vi "OTECCM-SECCM-Master-Program.vi"() -> ()   [LabVIEW 2016]
uses:
  SpectroElectroChem_1Electrode_caseEnum.ctl
  <vilib>/Utility/error.llb/DialogType.ctl
  <vilib>/DAQmx/write.llb/DAQmx Write (Analog 1D DBL 1Chan NSamp).vi
  <vilib>/DAQmx/write.llb/DAQmx Write (Analog DBL 1Chan 1Samp).vi
  <vilib>/DAQmx/read.llb/DAQmx Read (Analog 2D DBL NChan NSamp).vi
  <vilib>/Analysis/baseanly.llb/Mean (DBL).vi
  <vilib>/DAQmx/create/channels.llb/DAQmx Create Channel (AI-Voltage-Basic).vi
  <vilib>/DAQmx/configure/timing.llb/DAQmx Timing (Sample Clock).vi
  <vilib>/DAQmx/create/channels.llb/DAQmx Create Channel (AO-Voltage-Basic).vi
  <vilib>/DAQmx/miscellaneous.llb/DAQmx Fill In Error Info.vi
  <vilib>/Utility/file.llb/Write Delimited Spreadsheet (DBL).vi
  <vilib>/DAQmx/configure/trigger.llb/DAQmx Start Trigger (Digital Edge).vi
  <vilib>/Utility/file.llb/Write Delimited Spreadsheet (I64).vi
  <vilib>/DAQmx/configure/trigger.llb/DAQmx Start Trigger (None).vi
  <vilib>/measure/NI_MABase.lvlib
  <vilib>/Analysis/NI_AALBase.lvlib
  <resource>/objmgr/daqmx.rc
panel:
  out "dy":dbl
  out "ny":dbl
  out "dx":dbl
  out "nx":dbl
  in  "Clear POI":bool
  out "Points of Interest":dbl[][](array[numeric])
  out "Piezo Velocity / um/s":dbl[](array[numeric]) format="%.6f"
  out "Stopped":bool
  out "Piezo z":dbl
  out "Piezo y":dbl
  out "Piezo x":dbl
  out "Econtrol":refnum<k21>
  out "i tip":dbl(graph)
  out "E-Chem Data Point":i32
  in  "Stop Action":bool
  out "Acquisition Progress":u8(slide) scale=0.0..100.0
  out "Stage Task":refnum<k21>
  out "CCD Image":i32[][](graph)
  out "Background":i32[][](array[numeric])
  in  "Tab Control":T1(tab)
  in  "Tip Filter (Hz)":u16(ring) items=["100", "300", "1K", "3K", "10K"]
  in  "Tip Gain (mV/pA)":dbl(ring)=1.0 items=["0.1"=0.1, "0.2"=0.2, "0.5"=0.5, "1"=1.0, "2"=2.0, "5"=5.0, "10"=10.0, "20"=20.0]
  in  "Cycles":dbl
  in  "Start CV":bool
  in  "Initial E / V":dbl
  in  "Final E / V":dbl
  in  "v / mV/s":dbl
  out "Tip Voltammogram":cluster{dbl[], dbl[]}(graph)
  in  "Setpoint Direction":u16(ring) items=["Positive", "Negative"]
  in  "Setpoint / A":dbl
  out "Tip Approach Curve":cluster{dbl[], dbl[]}(graph)
  in  "Initial z":dbl
  in  "Final z":dbl
  in  "z Res.":dbl
  in  "t / pt / s":dbl
  in  "Start Approach Curve":bool
  in  "Stop Approach \nCurve":bool
  in  "Stop TarSECCM":bool
  in  "Targeted SECCM":bool
  in  "Retraction / um":dbl=3.0
  in  "Approach Set / A":dbl=3e-12
  in  "E Approach / V":dbl=-0.75
  in  "t / s/pt":dbl=0.002
  in  "z Res. / um":dbl=0.004
  out "Height Image":dbl[][](graph)
  out "SECM Image":dbl[][](graph)
  in  "xi / um":dbl
  in  "xf / um":dbl=20.0
  in  "xy Res. / um":dbl=0.5
  in  "yi / um":dbl
  in  "yf / um":dbl=20.0
  in  "Start SECM Image":bool
  in  "Stop SECM Image":bool
  out "Tip Voltammogram 2":cluster{dbl[], dbl[]}(graph)
  out "Tip Approach Curve 2":cluster{dbl[], dbl[]}(graph)
  in  "SECCM SP Dir":u16(ring)=1 items=["Positive", "Negative"]
  in  "CV v / mV/s":dbl=2000.0
  in  "CV Ef / V":dbl=0.5
  in  "CV Ei / V":dbl=-0.75
  in  "CV Cycles":dbl=0.5
  in  "Clear Background":bool
  in  "Aquire Background":bool
  out "xpixels":i32
  out "ypixels":i32
  in  "HSS (MHz)":i32(ring) items=["3.000000", "1.000000", "0.050000"]
  in  "VSS (us)":i32(ring) items=["4.880000", "9.680000", "19.280001", "38.470001", "57.680000"]
  in  "Exp. Time":sgl=0.1 format="%.2f"
  in  "# of Acc.":i32=1
  in  "EM Gain":i32=1
  in  "Binning":i32=1
  out "Cycle Time":sgl format="%.2f"
  out "Actual Temp.":i32
  in  "Background \nFrames":i32=10
  in  "Slit Width (um)":dbl=50.0
  in  "Center Wavelength (nm)":dbl
  out "Left":dbl
  out "Center":dbl
  out "Right":dbl
  in  "Grating":u16(ring) items=["1", "2", "3"]
  out "Lines/mm":i32=300
  in  "x Step (um)":dbl=0.25
  in  "Final x (um)":dbl=20.0
  in  "Initial x (um)":dbl
  out "Total Intensity":i32[][](graph)
  in  "Rest x (um)":dbl
  in  "Get HSI":bool
  in  "Delta":dbl=0.9267
  in  "Gamma":dbl=-0.064
  in  "Beta":dbl=0.0061
  in  "Alpha":dbl=1.1435
  in  "y":dbl
  in  "y'":dbl
  in  "x'":dbl
  in  "x":dbl
  out "bx":dbl
  out "by":dbl
  in  "Sample z":dbl
  in  "Sample y":dbl
  in  "Sample x":dbl
  out "Piezo Axes":string[](array[string])
  out "Resting?":bool
  out "Monitor":refnum<k21>
  out "Etip":dbl(graph)
  in  "WE Rest E (V)":dbl=-0.75
  out "Cell On?":bool
  out "Connected?":bool
  in  "Shutdown":bool
  # "HSI"
  # "SECCM"
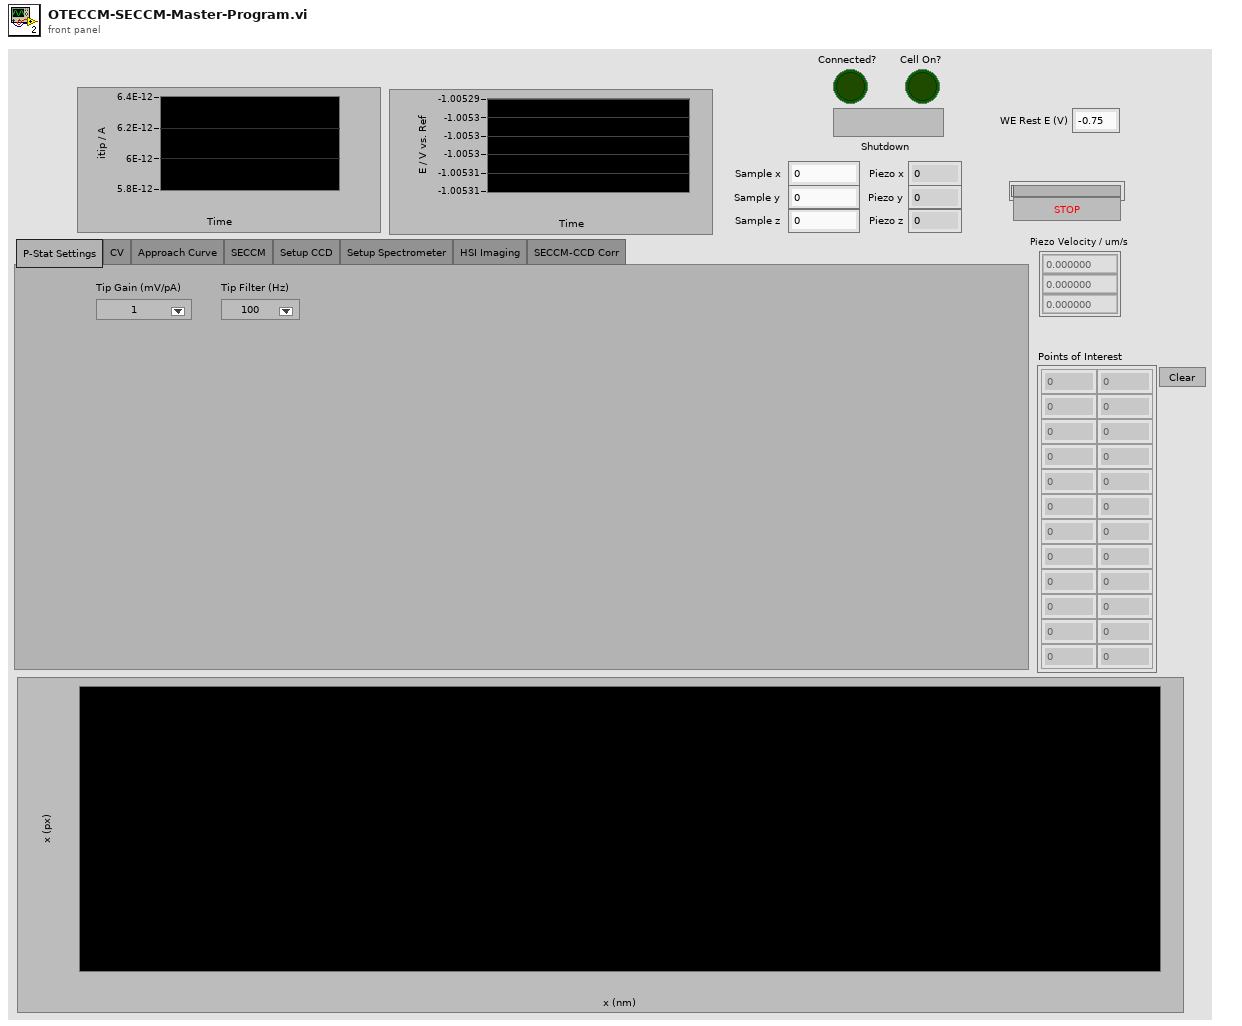
[diagram p1: front panel]
types:
  T1 = enum32{"P-Stat Settings", "CV", "Approach Curve", "SECCM", "Setup CCD", "Setup Spectrometer", "HSI Imaging", "SECCM-CCD Corr"}
  T2 = typedef "SpectroElectroChem_1Electrode_caseEnum.ctl" = enum16{"Initialize", "Rest", "Set Range", "Change Grating", "Move Grating", "Adjust Slit", "Setup CCD", "Acquire CCD BG", "Clear CCD BG", "Move Stage", "Cell On", "Cell Off", "Set E", "Move Piezo", "Acquire HSI", "Approach Curve", "Acquire SECCM Image", "Targeted SECCM", "Acquire CV", "Shutdown"}
  T3 = typedef "DialogType.ctl" = u16
  T4 = typedef "LVPoint32TypeDef.ctl" = cluster{"Horizontal":i32, "Vertical":i32}
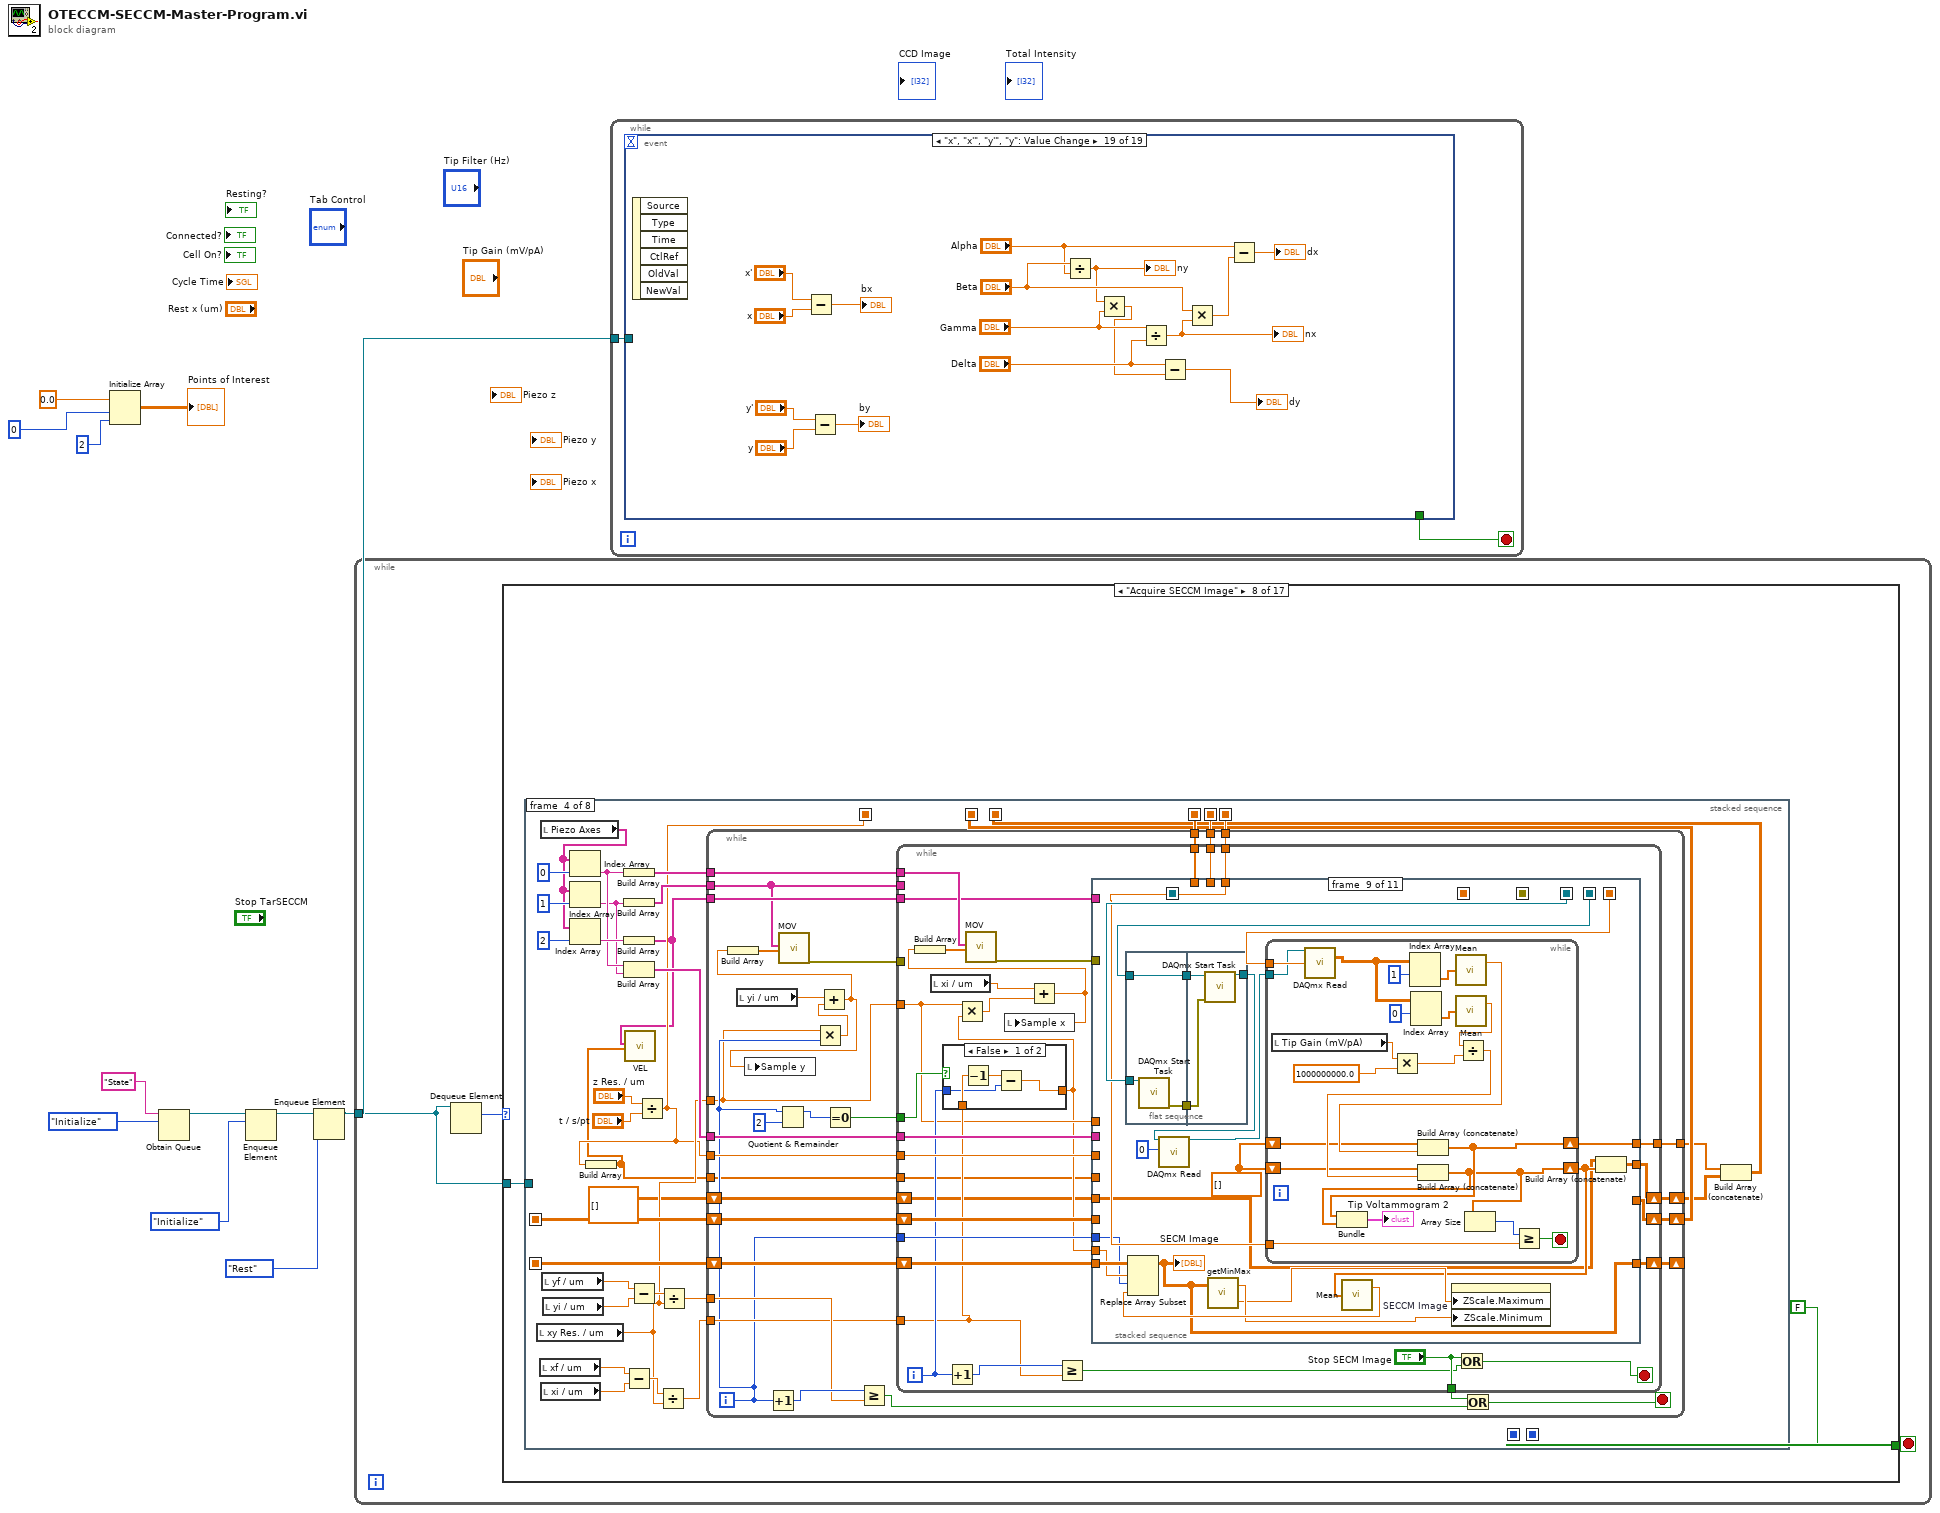
[diagram p0: block diagram]
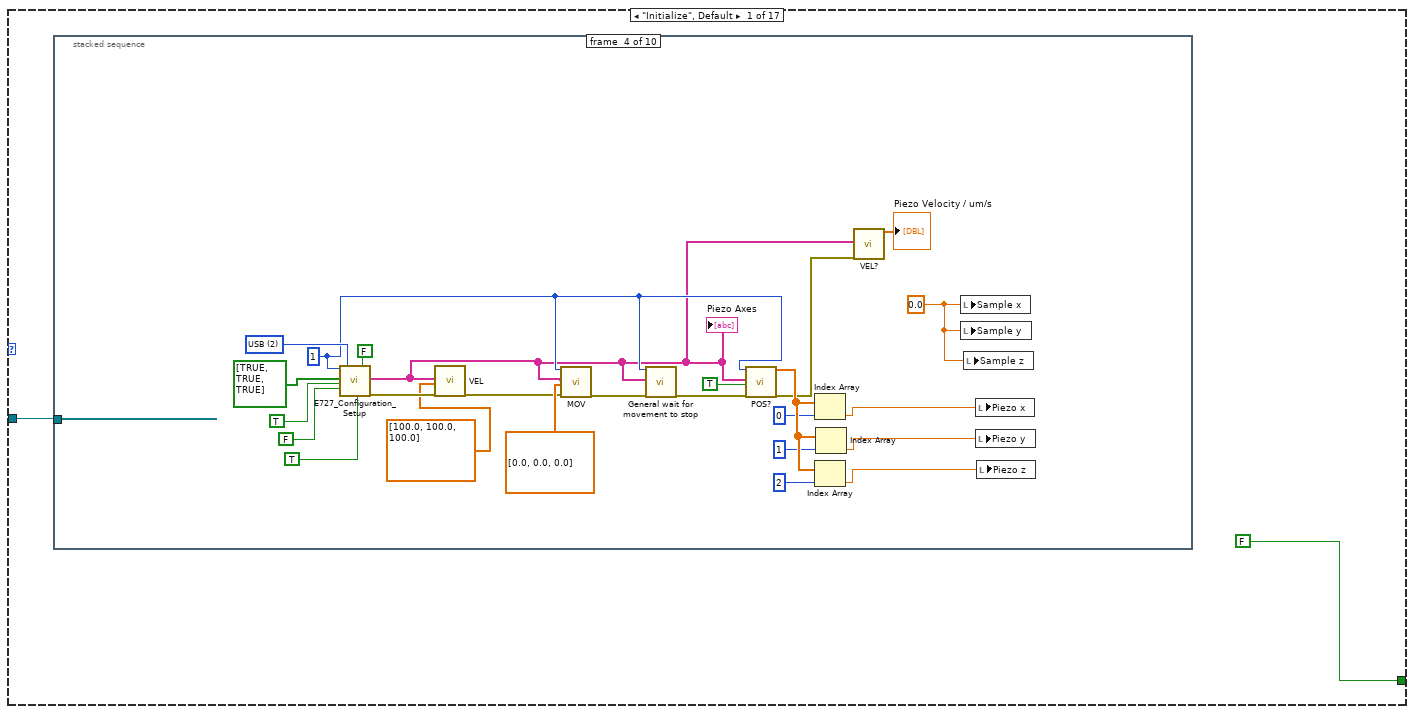
[diagram p2: hidden frame]
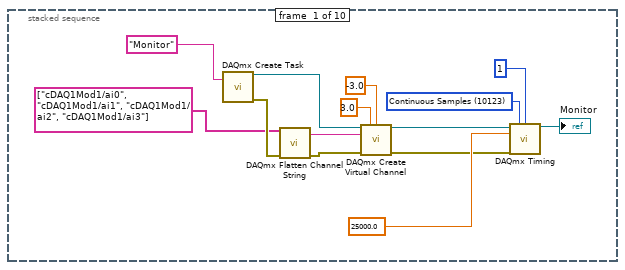
[diagram p3: hidden frame]
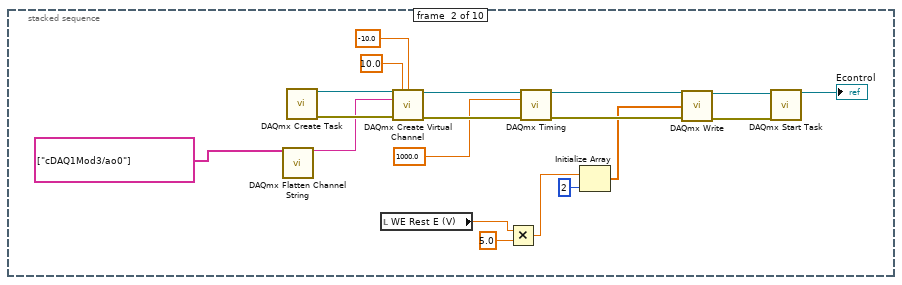
[diagram p4: hidden frame]
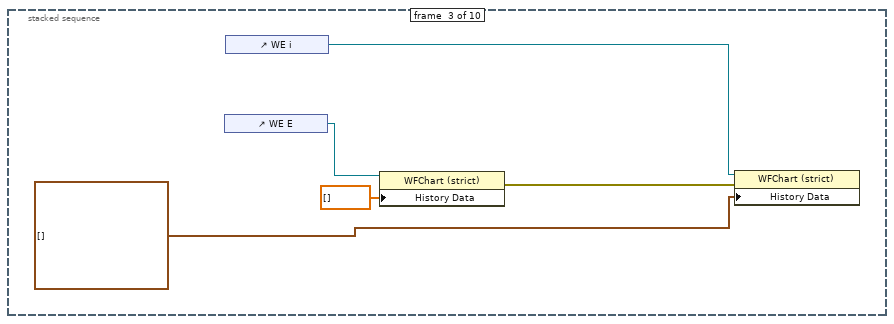
[diagram p5: hidden frame]
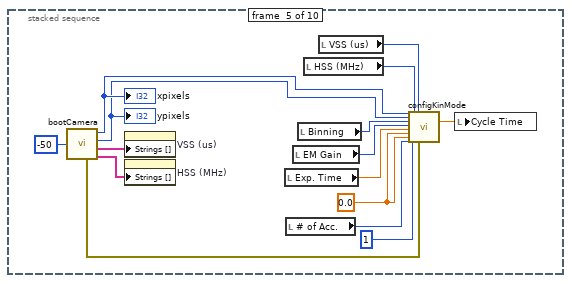
[diagram p6: hidden frame]
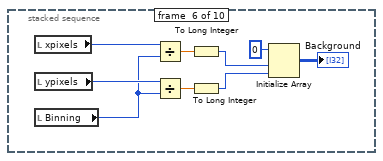
[diagram p7: hidden frame]
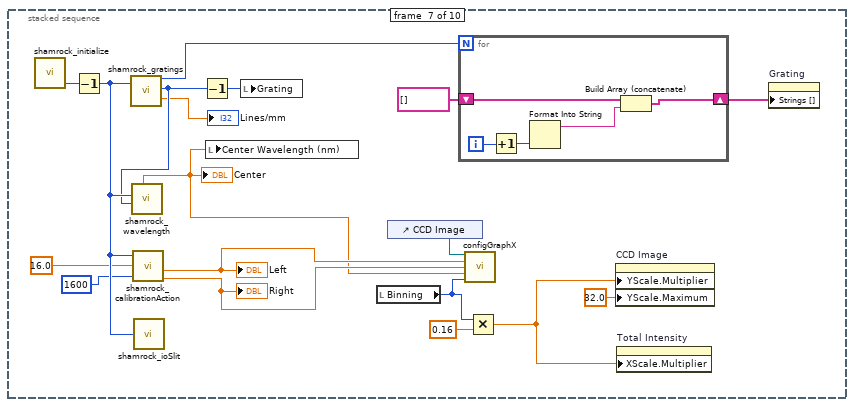
[diagram p8: hidden frame]
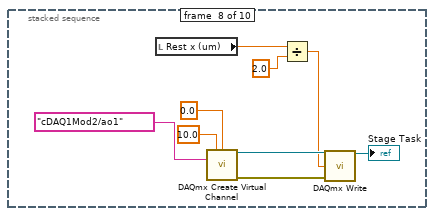
[diagram p9: hidden frame]
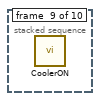
[diagram p10: hidden frame]
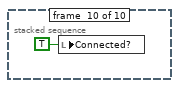
[diagram p11: hidden frame]
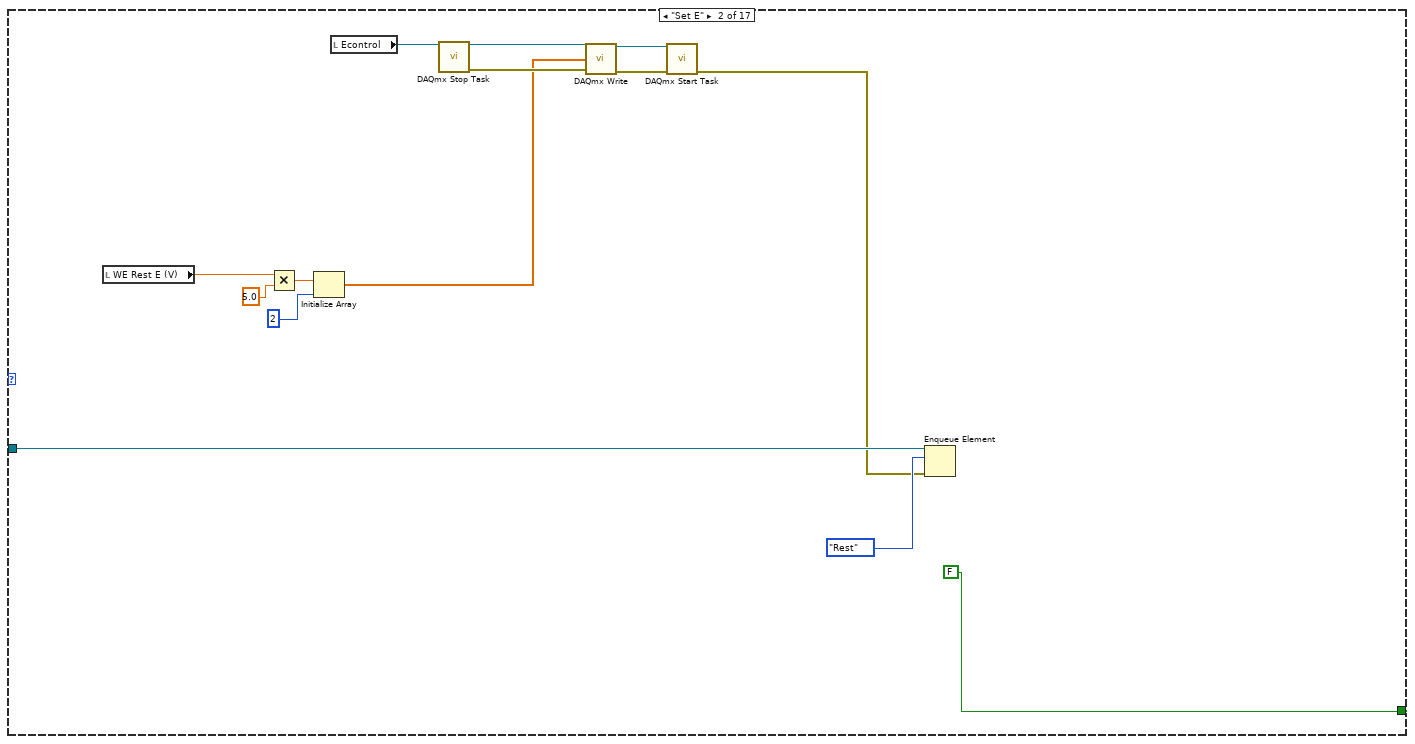
[diagram p12: hidden frame]
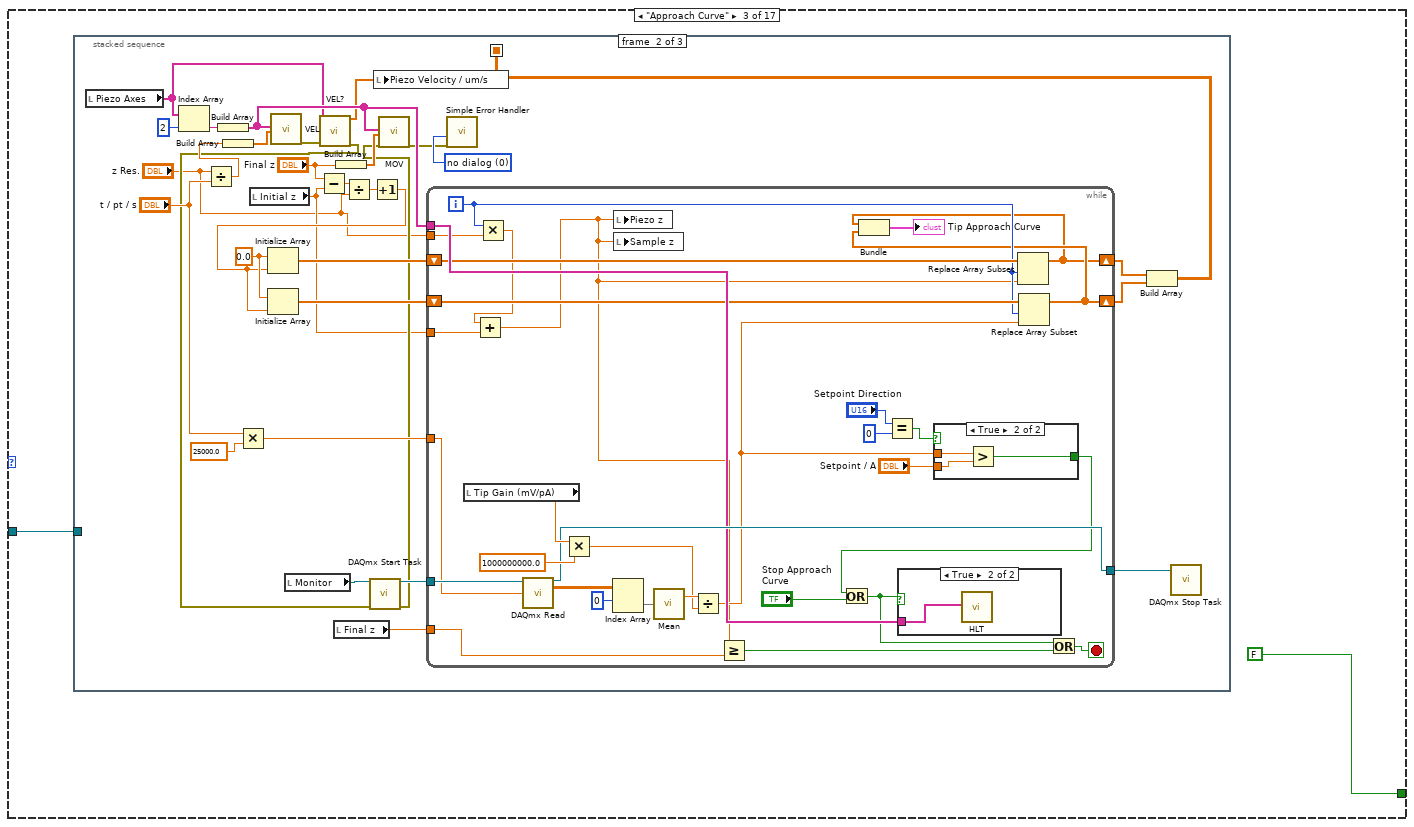
[diagram p13: hidden frame]
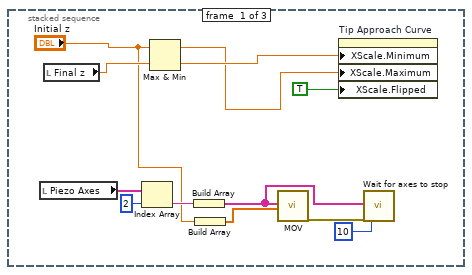
[diagram p14: hidden frame]
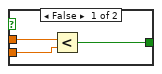
[diagram p15: hidden frame]
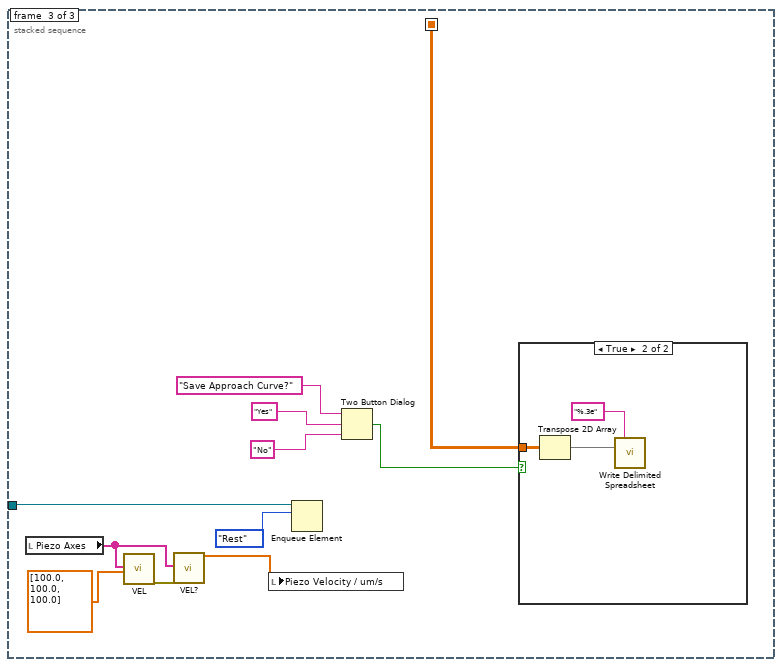
[diagram p17: hidden frame]
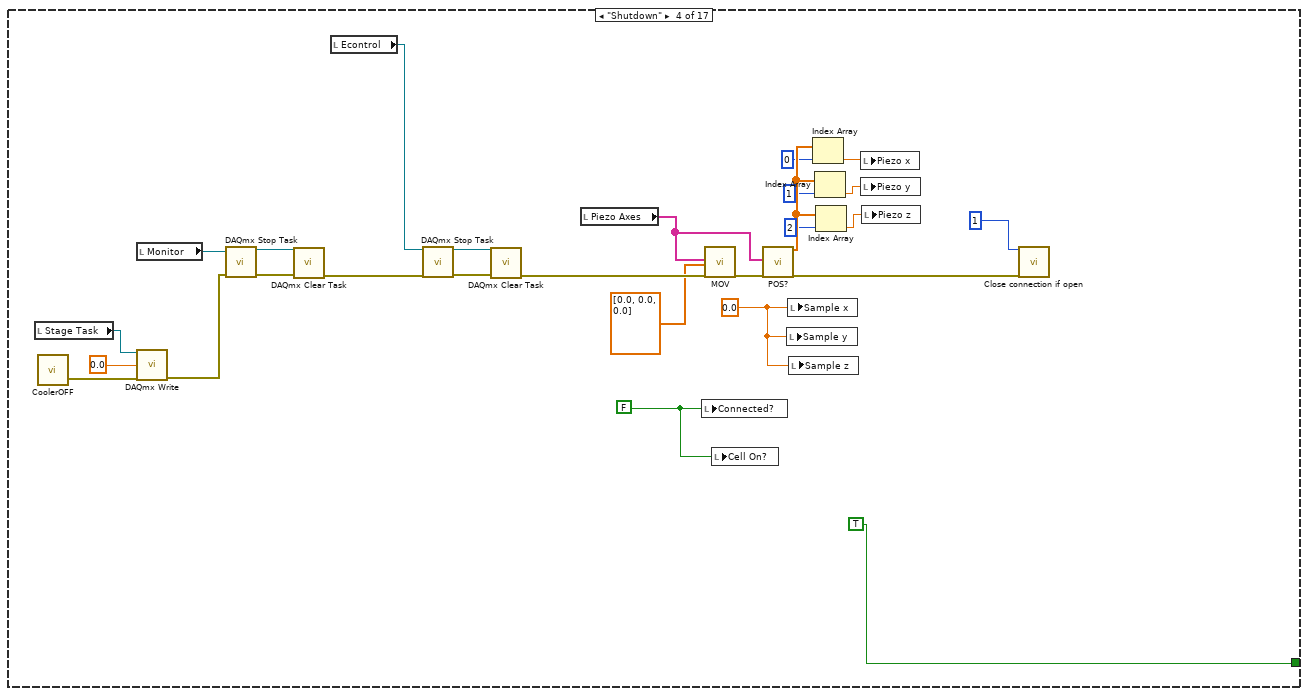
[diagram p19: hidden frame]
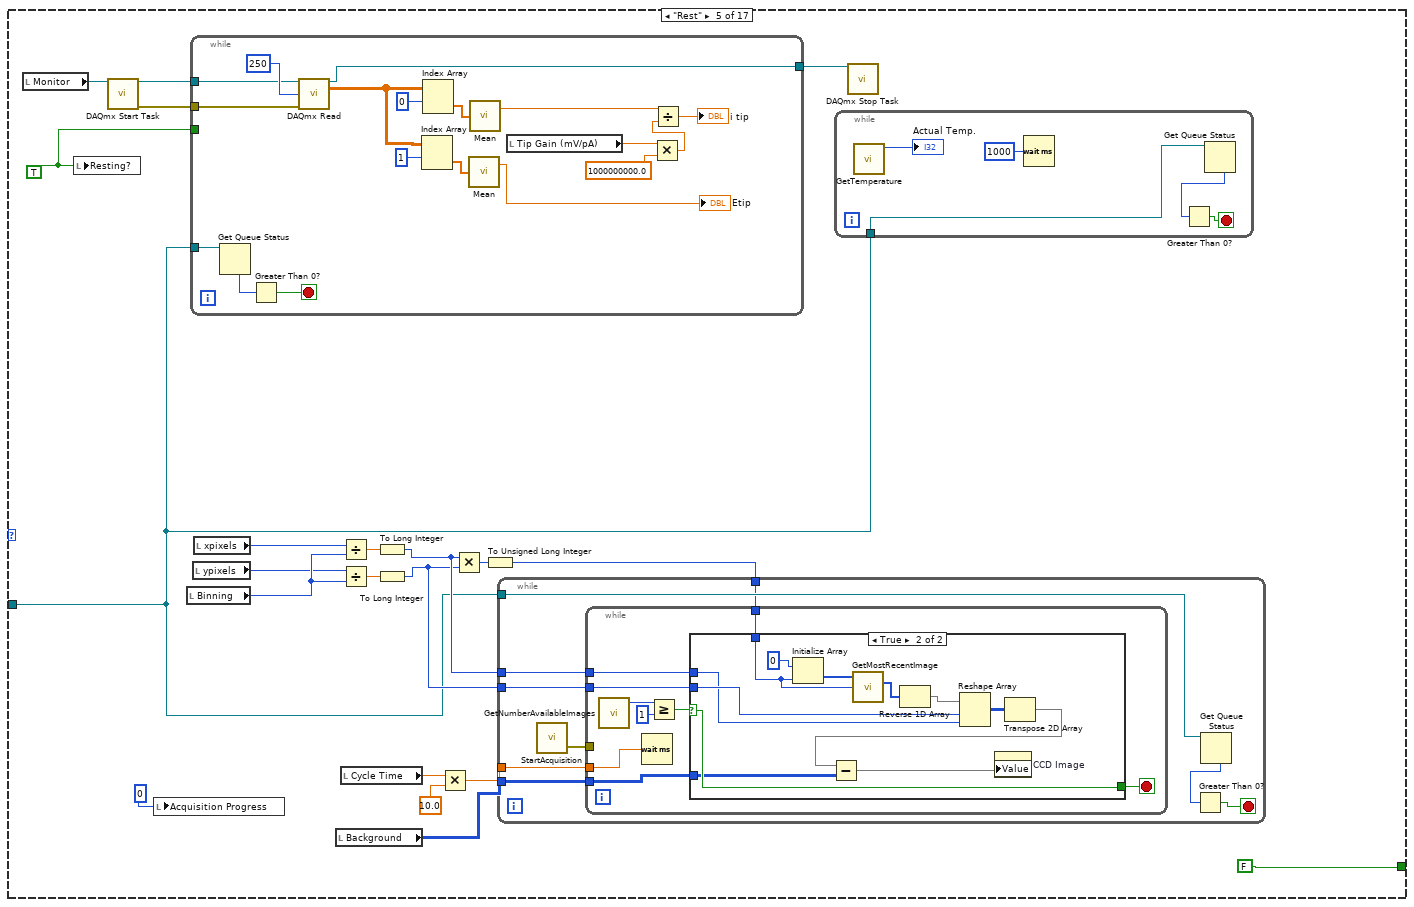
[diagram p20: hidden frame]
diagram:
  n1 = Initialize Array(0.0 ("element"), 0 ("dimension size"), 2 ("dimension size")) -> (→"Points of Interest":dbl[][])
  n2 = Obtain Queue(name (unnamed)="State", element data type=SpectroElectroChem_1Electrode_caseEnum."Initialize") -> (queue out=w10:refnum<queue>)  [unwired: 3 in, 2 out]
  n3 = Enqueue Element(queue=w10, element=SpectroElectroChem_1Electrode_caseEnum."Initialize") -> (queue out=w8:refnum<queue>)  [unwired: 2 in, 2 out]
  n4 = Enqueue Element(queue=w8, element=SpectroElectroChem_1Electrode_caseEnum."Rest") -> (queue out=w6:refnum<queue>)  [unwired: 2 in, 2 out]
  n5 = while {
    tunnel: w6 -> [w13]
    stop <- w14 stop-if-true
    n6 = Dequeue Element(queue=w13) -> (element=w12:T2)  [unwired: 2 in, 3 out]
    n7 = case shown="\"Acquire SECCM Image\"" w12 {
      tunnel: [FALSE FALSE FALSE TRUE FALSE FALSE FALSE FALSE FALSE FALSE FALSE FALSE FALSE FALSE FALSE FALSE FALSE] -> w14
      tunnel: w13 -> [w15 w143 w151 _ w279 w352 w381 w578 w1010 w1033 w1055 w1079 w1103 w1169 _ w1190 w1313]
      frame "Initialize", Default {
        n8 = stacked-sequence {
          tunnel: w15 -> [_ _ _ _ _ _ _ _ _ _]
          frame #0 {
            w21 = 10123 items=["Finite Samples"=10178, "Continuous Samples"=10123, "Hardware Timed Single Point"=12522] ("sample mode")
            n9 = call <vilib>:"DAQmx Create Task.vi"("new task name"="Monitor") -> ("task out"=w26:refnum<k21>, "error out"=w27:errorcluster)  [unwired: 13 in]
            n10 = call <vilib>:"DAQmx Flatten Channel String.vi"("names in"=tag[] ["cDAQ1Mod1/ai0", "cDAQ1Mod1/ai1", "cDAQ1Mod1/ai2", "cDAQ1Mod1/ai3"] ("physical channels"), "error in"=w27) -> ("names out"=w29:string, "error out"=w28:errorcluster)  [unwired: 12 in]
            n11 = call-poly <vilib>:"DAQmx Create Virtual Channel.vi"("task in"=w26, "maximum value"=3.0, "minimum value"=-3.0, "physical channels"=w29, "error in"=w28) -> ("task out"=w24:refnum<k21>, "error out"=w22:errorcluster)  [unwired: 9 in]
            n12 = call-poly <vilib>:"DAQmx Timing.vi"("task/channels in"=w24, "sample mode"=w21, "samples per channel"=1, "rate"=25000.0, "error in"=w22) -> ("task out"=→"Monitor":refnum<k21>)  [unwired: 9 in, 1 out]
          }
          frame #1 {
            n13 = call <vilib>:"DAQmx Flatten Channel String.vi"("names in"=tag[] ["cDAQ1Mod3/ao0"] ("physical channels")) -> ("names out"=w33:string)  [unwired: 13 in, 1 out]
            n14 = call <vilib>:"DAQmx Create Task.vi"() -> ("task out"=w49:refnum<k21>, "error out"=w43:errorcluster)  [unwired: 14 in]
            n15 = local read "WE Rest E (V)"() -> (w32:dbl)
            n16 = call-poly <vilib>:"DAQmx Create Virtual Channel.vi"("task in"=w49, "maximum value"=10.0, "minimum value"=-10.0, "physical channels"=w33, "error in"=w43) -> ("task out"=w48:refnum<k21>, "error out"=w42:errorcluster)  [unwired: 9 in]
            n17 = Multiply(x=w32, y=5.0) -> (x*y=w35:dbl)
            n18 = call-poly <vilib>:"DAQmx Timing.vi"("task/channels in"=w48, "rate"=1000.0, "error in"=w42) -> ("task out"=w47:refnum<k21>, "error out"=w41:errorcluster)  [unwired: 11 in]
            n19 = Initialize Array(w35, 2 ("dimension size")) -> (w31:dbl[])
            n20 = call-poly <vilib>:"DAQmx Write.vi"("task/channels in"=w47, "data"=w31, "error in"=w41) -> ("task out"=w46:refnum<k21>, "error out"=w40:errorcluster)  [unwired: 10 in, 1 out]
            n21 = call <vilib>:"DAQmx Start Task.vi"("task/channels in"=w46, "error in"=w40) -> ("task out"=→"Econtrol":refnum<k21>)  [unwired: 12 in, 1 out]
          }
          frame #2 {
            n22 = control-ref of="WE E"() -> (w54:refnum<vi>)
            n23 = control-ref of="WE i"() -> (w52:refnum<vi>)
            n24 = property on="Property Node" class="WFChart (strict)"(reference=w54, "History Data"=dbl[] []) -> (error out=w51:errorcluster)  [unwired: 1 in, 1 out]
            n25 = property on="Property Node" class="WFChart (strict)"(reference=w52, error in=w51, "History Data"=waveform(dbl)[] []) -> ()  [unwired: 2 out]
          }
          frame #3 {
            w55 = 0.0 ("Sample x")
            w62 = 1 ("System no.")
            w79 = u16 2 items=["RS232", "TCP/IP", "USB"] ("Interface")
            n26 = call "E727_Configuration_Setup.vi"("System no."=w62, "Are stages connected?"=bool[] [TRUE, TRUE, TRUE], "Change servo status to ON?"=TRUE, "Perform autozero?"=FALSE, "Interface"=w79, "Stop wave generator\noutput (if any)"=TRUE ("Stop wave generator\noutput (if any)"), "Move to middle?"=FALSE) -> ("All conn. axes"=w58:string[], "error out"=w61:errorcluster)  [unwired: 8 in, 3 out]
            "Piezo Axes" <- w58
            n27 = call "VEL.vi"("Axes to set"=w58, "Velocity values"=dbl[] [100.0, 100.0, 100.0] ("Position values"), "error in"=w61) -> ("error out"=w60:errorcluster)  [unwired: 15 in, 1 out]
            n28 = call "MOV.vi"("System no."=w62, "Axes to move"=w58, "Position values"=dbl[] [0.0, 0.0, 0.0], "error in"=w60) -> ("error out"=w71:errorcluster)  [unwired: 15 in]
            n29 = call "General wait for movement to stop.vi"("System no."=w62, "Axes to wait for"=w58, "error in"=w71) -> ("error out"=w70:errorcluster)  [unwired: 15 in, 1 out]
            n30 = call "POS?.vi"("System no."=w62, "Axes to query"=w58, "All axes?"=TRUE, "error in"=w70) -> ("Position"=w69:dbl[], "error out"=w57:errorcluster)  [unwired: 14 in]
            n31 = Index Array(array=w69, index=0) -> (element=w65:dbl)
            n32 = Index Array(array=w69, index=2) -> (element=w63:dbl)
            n33 = Index Array(array=w69, index=1) -> (element=w64:dbl)
            n34 = call "VEL?.vi"("Axes to query"=w58, "error in"=w57) -> ("Velocity"=→"Piezo Velocity / um/s":dbl[])  [unwired: 16 in, 1 out]
            n35 = local write "Sample x"(w55) -> ()
            n36 = local write "Sample y"(w55) -> ()
            n37 = local write "Sample z"(w55) -> ()
            n38 = local write "Piezo x"(w65) -> ()
            n39 = local write "Piezo y"(w64) -> ()
            n40 = local write "Piezo z"(w63) -> ()
          }
          frame #4 {
            w86 = sgl 0.0 ("Acc. Cycle Time")
            n41 = call "bootCamera.vi"("Target Temp"=-50) -> ("xpixels"=w81:i32, "ypixels"=w80:i32, "error out"=w83:errorcluster, "VSS"=w93:string[], "HSS"=w92:string[])  [unwired: 5 in]
            "xpixels" <- w81
            "ypixels" <- w80
            n42 = property on="VSS (us)" class="Ring (strict)"("Strings []"=w93) -> ()  [unwired: 2 in, 2 out]
            n43 = property on="HSS (MHz)" class="Ring (strict)"("Strings []"=w92) -> ()  [unwired: 2 in, 2 out]
            n44 = local read "Exp. Time"() -> (w87:sgl)
            n45 = local read "# of Acc."() -> (w85:i32)
            n46 = local read "EM Gain"() -> (w88:i32)
            n47 = local read "Binning"() -> (w89:i32)
            n48 = local read "HSS (MHz)"() -> (w90:i32)
            n49 = local read "VSS (us)"() -> (w91:i32)
            n50 = call "configKinMode.vi"("X Pixels"=w81, "Y Pixels"=w80, "Binning"=w89, "EM Gain"=w88, "Exp. Time"=w87, "Acc. Cycle Time"=w86, "Kin. Cycle Time"=w86, "# of Acc."=w85, "HSS"=w90, "# of Scans"=1, "VSS"=w91, "error in (no error)"=w83) -> ("Actual Kin. Cycle Time"=w82:sgl)  [unwired: 12 in, 3 out]
            n51 = local write "Cycle Time"(w82) -> ()
          }
          frame #5 {
            n52 = local read "xpixels"() -> (w97:i32)
            n53 = local read "ypixels"() -> (w96:i32)
            n54 = local read "Binning"() -> (w95:i32)
            n55 = Divide(x=w97, y=w95) -> (x/y=w103:dbl)
            n56 = Divide(x=w96, y=w95) -> (x/y=w102:dbl)
            n57 = To Long Integer(number=w103) -> (32bit integer=w100:i32)
            n58 = To Long Integer(number=w102) -> (32bit integer=w99:i32)
            n59 = Initialize Array(0 ("element"), w100, w99) -> (→"Background":i32[][])
          }
          frame #6 {
            n60 = call "shamrock_initialize.vi"() -> ("No of devices"=w121:i32)  [unwired: 1 in, 2 out]
            n61 = Decrement(x=w121) -> (x-1=w120:i32)
            n62 = call "shamrock_gratings.vi"("Device No"=w120) -> ("No Gratings"=w112:i32, "Grating"=w116:i32, "lines/mm"=→"Lines/mm":dbl)  [unwired: 1 in, 15 out]
            n63 = call "shamrock_wavelength.vi"("Grating No"=w116, "Device No"=w120) -> ("Wavelength"=w108:dbl)  [unwired: 8 out]
            "Center" <- w108
            n64 = call "shamrock_calibrationAction.vi"("Device No"=w120, "Set Pixel Width"=sgl 16.0, "Set Number Pixels"=1600) -> ("Wavelength First Pixel"=w110:sgl, "Wavelength Last Pixel"=w109:sgl)  [unwired: 3 out]
            "Left" <- w110
            "Right" <- w109
            n65 = call "shamrock_ioSlit.vi"("Device No"=w120) -> ()  [unwired: 8 out]
            n66 = Decrement(x=w116) -> (x-1=w117:i32)
            n67 = local write "Center Wavelength (nm)"(w108) -> ()
            n68 = local write "Grating"(w117) -> ()
            n69 = local read "Binning"() -> (w106:i32)
            n70 = control-ref of="CCD Image"() -> (w111:refnum<vi>)
            n71 = for {
              N: w112 -> [_]
              shift-right: [w124] -> w113
              shift-left: string[] [] -> [w126]
              i -> [w123]
              n72 = Increment(x=w123) -> (x+1=w122:i32)
              n73 = Format Into String(w122) -> (resulting string=w125:string)  [unwired: 3 in, 1 out]
              n74 = Build Array (concatenate)(w126, w125) -> (w124:string[])
            }
            n75 = call "configGraphX.vi"("Graph"=w111, "min"=w110, "max"=w109, "Center"=w108, "Binning"=w106) -> ()  [unwired: 11 in]
            n76 = Multiply(x=w106, y=0.16) -> (x*y=w104:dbl)
            n77 = property on="CCD Image" class="IntGraph (strict)"("YScale.Multiplier"=w104, "YScale.Maximum"=32.0 ("Y Scale.Range:Maximum")) -> ()  [unwired: 2 in, 2 out]
            n78 = property on="Total Intensity" class="IntGraph (strict)"("XScale.Multiplier"=w104) -> ()  [unwired: 2 in, 2 out]
            n79 = property on="Grating" class="Ring (strict)"("Strings []"=w113) -> ()  [unwired: 2 in, 2 out]
          }
          frame #7 {
            n80 = local read "Rest x (um)"() -> (w129:dbl)
            n81 = call-poly <vilib>:"DAQmx Create Virtual Channel.vi"("maximum value"=10.0, "minimum value"=0.0, "physical channels"=tag "cDAQ1Mod2/ao1") -> ("task out"=w132:refnum<k21>, "error out"=w131:errorcluster)  [unwired: 11 in]
            n82 = Divide(x=w129, y=2.0) -> (x/y=w127:dbl)
            n83 = call-poly <vilib>:"DAQmx Write.vi"("task/channels in"=w132, "data"=w127, "error in"=w131) -> ("task out"=→"Stage Task":refnum<k21>)  [unwired: 10 in, 2 out]
          }
          frame #8 {
            n84 = call <userlib>:"CoolerON.vi"() -> ()  [unwired: 2 in, 2 out]
          }
          frame #9 {
            n85 = local write "Connected?"(TRUE ("Connected?")) -> ()
          }
        }
      }
      frame "Set E" {
        n86 = local read "WE Rest E (V)"() -> (w138:dbl)
        n87 = Multiply(x=w138, y=5.0) -> (x*y=w141:dbl)
        n88 = Initialize Array(w141, 2 ("dimension size")) -> (w137:dbl[])
        n89 = local read "Econtrol"() -> (w149:refnum<k21>)
        n90 = call <vilib>:"DAQmx Stop Task.vi"("task/channels in"=w149) -> ("task out"=w148:refnum<k21>, "error out"=w145:errorcluster)  [unwired: 13 in]
        n91 = call-poly <vilib>:"DAQmx Write.vi"("task/channels in"=w148, "data"=w137, "error in"=w145) -> ("task out"=w147:refnum<k21>, "error out"=w146:errorcluster)  [unwired: 10 in, 1 out]
        n92 = call <vilib>:"DAQmx Start Task.vi"("task/channels in"=w147, "error in"=w146) -> ("error out"=w139:errorcluster)  [unwired: 12 in, 1 out]
        n93 = Enqueue Element(queue=w143, element=SpectroElectroChem_1Electrode_caseEnum."Rest", error in (no error)=w139) -> ()  [unwired: 1 in, 3 out]
      }
      frame "Approach Curve" {
        n94 = stacked-sequence {
          seq-local: [_ w185 _] -> [_ _ w240]
          tunnel: w151 -> [_ _ w246]
          frame #0 {
            n95 = local read "Piezo Axes"() -> (w160:string[])
            n96 = local read "Final z"() -> (w163:dbl)
            n97 = Index Array(array=w160, index=2) -> (element=w158:string)
            n98 = Max & Min(x="Initial z", y=w163) -> (max(x,y)=w161:dbl, min(x,y)=w162:dbl)
            n99 = Build Array(w158) -> (w155:string[])
            n100 = Build Array("Initial z") -> (w157:dbl[])
            n101 = call "MOV.vi"("Axes to move"=w155, "Position values"=w157) -> ("error out"=w154:errorcluster)  [unwired: 17 in]
            n102 = property on="Tip Approach Curve" class="XYGraph (strict)"("XScale.Minimum"=w162, "XScale.Maximum"=w161, "XScale.Flipped"=TRUE ("X Scale.Flipped")) -> ()  [unwired: 2 in, 2 out]
            n103 = call "Wait for axes to stop.vi"("Axes to wait for"=w155, "error in"=w154, "Polling cycle time, ms"=u32 10) -> ()  [unwired: 15 in, 2 out]
          }
          frame #1 {
            w174 = 0.0 ("element")
            w184 = T3 0 items=["no dialog", "OK message", "continue or stop message", "OK message + warnings", "continue/stop + warnings"] ("type of dialog (OK msg:1)")
            n104 = local read "Piezo Axes"() -> (w183:string[])
            n105 = Index Array(array=w183, index=2) -> (element=w195:string)
            n106 = Divide(x="z Res.", y="t / pt / s") -> (x/y=w194:dbl)
            n107 = Build Array(w195) -> (w191:string[])
            n108 = Build Array(w194) -> (w193:dbl[])
            n109 = Multiply(x="t / pt / s", y=25000.0) -> (x*y=w181:dbl)
            n110 = local read "Initial z"() -> (w166:dbl)
            n111 = call "VEL.vi"("Axes to set"=w191, "Velocity values"=w193) -> ("error out"=w179:errorcluster)  [unwired: 16 in, 1 out]
            n112 = local read "Monitor"() -> (w189:refnum<k21>)
            n113 = Subtract(x="Final z", y=w166) -> (x-y=w176:dbl)
            n114 = call "VEL?.vi"("Axes to query"=w183, "error in"=w179) -> ("Velocity"=w182:dbl[], "error out"=w167:errorcluster)  [unwired: 16 in]
            n115 = local read "Final z"() -> (w192:dbl)
            n116 = Build Array("Final z") -> (w190:dbl[])
            n117 = Divide(x=w176, y="z Res.") -> (x/y=w175:dbl)
            n118 = call <vilib>:"DAQmx Start Task.vi"("task/channels in"=w189, "error in"=w167) -> ("task out"=w188:refnum<k21>, "error out"=w168:errorcluster)  [unwired: 12 in]
            n119 = Increment(x=w175) -> (x+1=w173:dbl)
            n120 = Initialize Array(w174, w173) -> (w172:dbl[])
            n121 = Initialize Array(w174, w173) -> (w171:dbl[])
            n122 = local write "Piezo Velocity / um/s"(w182) -> ()
            n123 = call "MOV.vi"("Axes to move"=w191, "Position values"=w190, "error in"=w168) -> ("error out"=w178:errorcluster)  [unwired: 16 in]
            n124 = while {
              tunnel: w191 -> [w216]
              tunnel: w192 -> [w228]
              tunnel: w188 -> [w227]
              tunnel: [w219] -> w186
              tunnel: w181 -> [w204]
              shift-right: [w198] -> w169
              shift-left: w171 -> [w206]
              shift-right: [w197] -> w170
              shift-left: w172 -> [w207]
              tunnel: w166 -> [w203]
              tunnel: "z Res." -> [w201]
              i -> [w202]
              stop <- w217 stop-if-true
              n125 = local read "Tip Gain (mV/pA)"() -> (w221:dbl)
              n126 = Multiply(x=w202, y=w201) -> (x*y=w200:dbl)
              n127 = Add(x=w200, y=w203) -> (x+y=w199:dbl)
              n128 = call-poly <vilib>:"DAQmx Read.vi"("task/channels in"=w227, "number of samples per channel"=w204) -> ("task out"=w219:refnum<k21>, "data"=w222:dbl[][])  [unwired: 11 in, 1 out]
              n129 = Multiply(x=w221, y=1000000000.0) -> (x*y=w220:dbl)
              n130 = Index Array(array=w222, index (row)=0) -> (element=w225:dbl[])  [unwired: 1 in]
              n131 = local write "Piezo z"(w199) -> ()
              n132 = local write "Sample z"(w199) -> ()
              n133 = call-poly <vilib>:"Mean.vi"("X"=w225) -> ("mean"=w224:dbl)  [unwired: 1 out]
              n134 = Divide(x=w224, y=w220) -> (x/y=w205:dbl)
              n135 = Greater Or Equal?(x=w199, y=w228) -> (x >= y?=w218:bool)
              n136 = Equal?(x="Setpoint Direction", y=u16 0) -> (x = y?=w212:bool)
              n137 = case shown="True" w212 {
                tunnel: "Setpoint / A" -> [w230 w233]
                tunnel: w205 -> [w231 w234]
                tunnel: [w229 w232] -> w210
                frame False {
                  n138 = Less?(x=w231, y=w230) -> (x < y?=w229:bool)
                }
                frame True {
                  n139 = Greater?(x=w234, y=w233) -> (0:w232:bool)
                }
              }
              n140 = Or(x=w210, y="Stop Approach \nCurve") -> (x .or. y?=w209:bool)
              n141 = case shown="True" w209 {
                tunnel: w216 -> [_ w235]
                frame False {
                }
                frame True {
                  n142 = call "HLT.vi"("Affected axes"=w235) -> ()  [unwired: 18 in, 1 out]
                }
              }
              n143 = Replace Array Subset(array=w207, new element=w199, index=w202) -> (w197:dbl[])
              n144 = Replace Array Subset(array=w206, new element=w205, index=w202) -> (w198:dbl[])
              n145 = Bundle(w197, w198) -> (→"Tip Approach Curve":cluster{dbl[], dbl[]})  [unwired: 1 in]
              n146 = Or(x=w209, y=w218) -> (x .or. y?=w217:bool)
            }
            n147 = call <vilib>:"Simple Error Handler.vi"("type of dialog (OK msg:1)"=w184, "error in (no error)"=w178) -> ()  [unwired: 3 in, 5 out]
            n148 = Build Array(w170, w169) -> (w185:dbl[][])
            n149 = call <vilib>:"DAQmx Stop Task.vi"("task/channels in"=w186) -> ()  [unwired: 13 in, 2 out]
          }
          frame #2 {
            n150 = local read "Piezo Axes"() -> (w237:string[])
            n151 = call "VEL.vi"("Axes to set"=w237, "Velocity values"=dbl[] [100.0, 100.0, 100.0]) -> ("error out"=w238:errorcluster)  [unwired: 16 in, 1 out]
            n152 = call "VEL?.vi"("Axes to query"=w237, "error in"=w238) -> ("Velocity"=w239:dbl[])  [unwired: 16 in, 1 out]
            n153 = local write "Piezo Velocity / um/s"(w239) -> ()
            n154 = Enqueue Element(queue=w246, element=SpectroElectroChem_1Electrode_caseEnum."Rest") -> ()  [unwired: 2 in, 3 out]
            n155 = Two Button Dialog(message="Save Approach Curve?", 1:"No" ("F button name (\"Cancel\")"), 2:"Yes" ("T button name (\"OK\")")) -> (T button?=w241:bool)
            n156 = case shown="True" w241 {
              tunnel: w240 -> [_ w249]
              frame False {
              }
              frame True {
                n157 = Transpose 2D Array(2D array=w249) -> (transposed array=w248:dbl[][])
                n158 = call-poly <vilib>:"Write Delimited Spreadsheet.vi"("format (%.3f)"="%.3e", "2D data"=w248) -> ()  [unwired: 12 in, 2 out]
              }
            }
          }
        }
      }
      frame "Shutdown" {
        w250 = 0.0 ("Sample x")
        w268 = FALSE ("Connected?")
        n159 = local read "Stage Task"() -> (w263:refnum<k21>)
        n160 = call <userlib>:"CoolerOFF.vi"() -> ("error out"=w265:errorcluster)  [unwired: 2 in, 1 out]
        n161 = local read "Monitor"() -> (w276:refnum<k21>)
        n162 = call-poly <vilib>:"DAQmx Write.vi"("task/channels in"=w263, "data"=0.0, "error in"=w265) -> ("error out"=w264:errorcluster)  [unwired: 10 in, 2 out]
        n163 = call <vilib>:"DAQmx Stop Task.vi"("task/channels in"=w276, "error in"=w264) -> ("task out"=w275:refnum<k21>, "error out"=w274:errorcluster)  [unwired: 12 in]
        n164 = call <vilib>:"DAQmx Clear Task.vi"("task in"=w275, "error in"=w274) -> ("error out"=w269:errorcluster)  [unwired: 13 in]
        n165 = local read "Econtrol"() -> (w270:refnum<k21>)
        n166 = call <vilib>:"DAQmx Stop Task.vi"("task/channels in"=w270, "error in"=w269) -> ("task out"=w272:refnum<k21>, "error out"=w271:errorcluster)  [unwired: 12 in]
        n167 = call <vilib>:"DAQmx Clear Task.vi"("task in"=w272, "error in"=w271) -> ("error out"=w262:errorcluster)  [unwired: 13 in]
        n168 = local read "Piezo Axes"() -> (w258:string[])
        n169 = local write "Connected?"(w268) -> ()
        n170 = call "MOV.vi"("Axes to move"=w258, "Position values"=dbl[] [0.0, 0.0, 0.0], "error in"=w262) -> ("error out"=w260:errorcluster)  [unwired: 16 in]
        n171 = local write "Cell On?"(w268) -> ()
        n172 = call "POS?.vi"("Axes to query"=w258, "error in"=w260) -> ("Position"=w257:dbl[], "error out"=w259:errorcluster)  [unwired: 16 in]
        n173 = local write "Sample y"(w250) -> ()
        n174 = local write "Sample x"(w250) -> ()
        n175 = local write "Sample z"(w250) -> ()
        n176 = Index Array(array=w257, index=0) -> (element=w253:dbl)
        n177 = Index Array(array=w257, index=1) -> (element=w252:dbl)
        n178 = Index Array(array=w257, index=2) -> (element=w251:dbl)
        n179 = local write "Piezo x"(w253) -> ()
        n180 = local write "Piezo y"(w252) -> ()
        n181 = local write "Piezo z"(w251) -> ()
        n182 = call "Close connection if open.vi"("System no."=1, "error in"=w259) -> ()  [unwired: 16 in, 2 out]
      }
      frame "Rest" {
        w294 = TRUE ("Resting?")
        n183 = local read "Monitor"() -> (w277:refnum<k21>)
        n184 = local write "Resting?"(w294) -> ()
        n185 = call <vilib>:"DAQmx Start Task.vi"("task/channels in"=w277) -> ("task out"=w296:refnum<k21>, "error out"=w297:errorcluster)  [unwired: 13 in]
        n186 = local write "Acquisition Progress"(u8 0 ("Acquisition Progress")) -> ()
        n187 = local read "Binning"() -> (w289:i32)
        n188 = while {
          tunnel: w296 -> [w350]
          tunnel: w297 -> [w349]
          tunnel: w294 -> [_]
          tunnel: [w348] -> w293
          tunnel: w279 -> [w347]
          stop <- w345 stop-if-true
          n189 = Get Queue Status(queue=w347) -> (# elements in queue=w346:i32)  [unwired: 2 in, 7 out]
          n190 = Greater Than 0?(x=w346) -> (x > 0?=w345:bool)
          n191 = call-poly <vilib>:"DAQmx Read.vi"("task/channels in"=w350, "number of samples per channel"=250, "error in"=w349) -> ("task out"=w348:refnum<k21>, "data"=w340:dbl[][])  [unwired: 10 in, 1 out]
          n192 = Index Array(array=w340, index (row)=1) -> (element=w342:dbl[])  [unwired: 1 in]
          n193 = Index Array(array=w340, index (row)=0) -> (element=w343:dbl[])  [unwired: 1 in]
          n194 = call-poly <vilib>:"Mean.vi"("X"=w342) -> ("mean"=→"Etip":dbl)  [unwired: 1 out]
          n195 = call-poly <vilib>:"Mean.vi"("X"=w343) -> ("mean"=w336:dbl)  [unwired: 1 out]
          n196 = local read "Tip Gain (mV/pA)"() -> (w339:dbl)
          n197 = Multiply(x=w339, y=1000000000.0) -> (x*y=w337:dbl)
          n198 = Divide(x=w336, y=w337) -> (x/y=→"i tip":dbl)
        }
        n199 = local read "ypixels"() -> (w285:i32)
        n200 = local read "xpixels"() -> (w284:i32)
        n201 = local read "Background"() -> (w282:i32[][])
        n202 = Divide(x=w284, y=w289) -> (x/y=w292:dbl)
        n203 = Divide(x=w285, y=w289) -> (x/y=w291:dbl)
        n204 = local read "Cycle Time"() -> (w288:sgl)
        n205 = To Long Integer(number=w292) -> (32bit integer=w281:i32)
        n206 = To Long Integer(number=w291) -> (32bit integer=w280:i32)
        n207 = Multiply(x=w288, y=sgl 10.0) -> (x*y=w286:sgl)
        n208 = Multiply(x=w281, y=w280) -> (x*y=w290:i32)
        n209 = To Unsigned Long Integer(number=w290) -> (unsigned 32bit integer=w283:u32)
        n210 = while {
          tunnel: w279 -> [w308]
          tunnel: w286 -> [w307]
          tunnel: w280 -> [w305]
          tunnel: w281 -> [w306]
          tunnel: w283 -> [w304]
          tunnel: w282 -> [w303]
          stop <- w309 stop-if-true
          n211 = call <userlib>:"StartAcquisition.vi"() -> ("error out"=w310:errorcluster)  [unwired: 2 in, 1 out]
          n212 = while {
            tunnel: w310 -> [_]
            tunnel: w307 -> [w316]
            tunnel: w306 -> [w315]
            tunnel: w305 -> [w314]
            tunnel: w304 -> [w313]
            tunnel: w303 -> [w312]
            stop <- w317 stop-if-true
            n213 = call <userlib>:"GetNumberAvailableImages.vi"() -> ("first"=w320:i32)  [unwired: 3 in, 3 out]
            n214 = Wait (ms)(milliseconds to wait=w316) -> ()  [unwired: 1 out]
            n215 = Greater Or Equal?(x=w320, y=1) -> (x >= y?=w318:bool)
            n216 = case shown="True" w318 {
              selector: w318 -> [w321 w327]
              tunnel: [w321 w327] -> w317
              tunnel: w315 -> [_ w324]
              tunnel: w314 -> [_ w325]
              tunnel: w313 -> [_ w326]
              tunnel: w312 -> [_ w323]
              frame False {
              }
              frame True {
                n217 = Initialize Array(0 ("element"), w326) -> (w332:i32[])
                n218 = call <userlib>:"GetMostRecentImage.vi"("size"=w326, "array"=w332) -> ("array"=w330:i32[])  [unwired: 1 in, 2 out]
                n219 = Reverse 1D Array(array=w330) -> (reversed array=w331:i32[])
                n220 = Reshape Array(w331, w325, w324) -> (w329:i32[][])
                n221 = Transpose 2D Array(2D array=w329) -> (transposed array=w328:i32[][])
                n222 = Subtract(x=w328, y=w323) -> (x-y=w322:i32[][])
                n223 = property on="CCD Image" class="IntGraph (strict)"("Value"=w322) -> ()  [unwired: 2 in, 2 out]
              }
            }
          }
          n224 = Get Queue Status(queue=w308) -> (# elements in queue=w311:i32)  [unwired: 2 in, 7 out]
          n225 = Greater Than 0?(x=w311) -> (x > 0?=w309:bool)
        }
        n226 = while {
          tunnel: w279 -> [w298]
          stop <- w299 stop-if-true
          n227 = call <userlib>:"GetTemperature.vi"() -> ("temperature"=→"Actual Temp.":i32)  [unwired: 4 in, 3 out]
          n228 = Wait (ms)(milliseconds to wait=u32 1000) -> ()  [unwired: 1 out]
          n229 = Get Queue Status(queue=w298) -> (# elements in queue=w300:i32)  [unwired: 2 in, 7 out]
          n230 = Greater Than 0?(x=w300) -> (x > 0?=w299:bool)
        }
        n231 = call <vilib>:"DAQmx Stop Task.vi"("task/channels in"=w293) -> ()  [unwired: 13 in, 2 out]
      }
      frame "Move Piezo" {
        n232 = stacked-sequence {
          tunnel: w352 -> [_ w379]
          frame #0 {
            w360 = 1 ("System no.")
            n233 = local read "Piezo Axes"() -> (w367:string[])
            n234 = local read "Sample y"() -> (w355:dbl)
            n235 = local read "Sample x"() -> (w356:dbl)
            n236 = local read "Sample z"() -> (w354:dbl)
            n237 = Index Array(array=w367, index=0) -> (element=w374:string)
            n238 = Index Array(array=w367, index=1) -> (element=w368:string)
            n239 = Index Array(array=w367, index=2) -> (element=w366:string)
            n240 = Build Array(w374, w368, w366) -> (w373:string[])
            n241 = Build Array(w356, w355, w354) -> (w376:dbl[])
            n242 = call "MOV.vi"("System no."=w360, "Axes to move"=w373, "Position values"=w376) -> ("error out"=w378:errorcluster)  [unwired: 16 in]
            n243 = call "General wait for movement to stop.vi"("System no."=w360, "Axes to wait for"=w373, "All axes?"=TRUE, "error in"=w378, "Polling cycle \ntime, ms"=u32 250 ("Polling cycle \ntime, ms")) -> ("Stopped"=→"Stopped":bool, "error out"=w377:errorcluster)  [unwired: 13 in]
            n244 = call "POS?.vi"("System no."=w360, "Axes to query"=w373, "error in"=w377) -> ("Position"=w364:dbl[])  [unwired: 15 in, 1 out]
            n245 = Index Array(array=w364, index=0) -> (element=w363:dbl)
            n246 = Index Array(array=w364, index=1) -> (element=w362:dbl)
            n247 = Index Array(array=w364, index=2) -> (element=w361:dbl)
            n248 = local write "Piezo x"(w363) -> ()
            n249 = local write "Piezo y"(w362) -> ()
            n250 = local write "Piezo z"(w361) -> ()
          }
          frame #1 {
            n251 = Enqueue Element(queue=w379, element=SpectroElectroChem_1Electrode_caseEnum."Rest") -> ()  [unwired: 2 in, 3 out]
          }
        }
      }
      frame "Acquire CV" {
        n252 = stacked-sequence {
          seq-local: [w406 _ _ _] -> [_ w415 _ _]
          seq-local: [_ w429 _ _] -> [_ _ w472 w572]
          seq-local: [_ w439 _ _] -> [_ _ w473 _]
          seq-local: ["v / mV/s" _ _ _] -> [_ w428 _ _]
          seq-local: [w395 _ _ _] -> [_ w427 w466 _]
          seq-local: [_ w430 _ _] -> [_ _ w467 _]
          seq-local: [_ _ w463 _] -> [_ _ _ w563]
          seq-local: [w386 _ _ _] -> [_ w425 _ _]
          seq-local: [_ w417 _ _] -> [_ _ w462 _]
          seq-local: [_ w418 _ _] -> [_ _ w461 _]
          seq-local: [_ w416 _ _] -> [_ _ w457 _]
          tunnel: w381 -> [_ _ w448 w573]
          frame #0 {
            n253 = Subtract(x="Final E / V", y="Initial E / V") -> (x-y=w400:dbl)
            n254 = Absolute Value(x=w400) -> (abs(x)=w412:dbl)
            n255 = Multiply(x=w412, y=2000.0) -> (x*y=w410:dbl)
            n256 = Divide(x="v / mV/s", y=w410) -> (x/y=w388:dbl)
            n257 = Divide(x="v / mV/s", y=w388) -> (x/y=w396:dbl)
            n258 = Add(x="Final E / V", y="Initial E / V") -> (x+y=w392:dbl)
            n259 = Multiply(x=w396, y="Cycles") -> (x*y=w395:dbl)
            n260 = Divide(x=w400, y=2.0) -> (x/y=w398:dbl)
            n261 = Bundle("v / mV/s"="v / mV/s", w395) -> (w409:cluster{"v / mV/s":dbl, dbl})  [unwired: 1 in]
            n262 = Divide(x=w392, y=2.0) -> (x/y=w390:dbl)
            n263 = call <vilib>:"Triangle Waveform.vi"("offset"=w390, "sampling info"=w409, "reset signal"=FALSE, "phase"=270.0, "amplitude"=w398, "frequency"=w388) -> ("signal out"=w405:waveform(dbl))  [unwired: 4 in, 1 out]
            n264 = Reciprocal(x=w388) -> (1/x=w387:dbl)
            n265 = Multiply(x=w387, y="Cycles") -> (x*y=w386:dbl)
            n266 = Unbundle By Name(w405) -> ("Y"=w406:dbl[])
            n267 = Max & Min(x="Final E / V", y="Initial E / V") -> (max(x,y)=w404:dbl, min(x,y)=w402:dbl)
            n268 = Add(x=w402, y=-0.05) -> (x+y=w383:dbl)
            n269 = Add(x=w404, y=0.05) -> (x+y=w384:dbl)
            n270 = property on="Tip Voltammogram" class="XYGraph (strict)"("XScale.Maximum"=w384, "XScale.Minimum"=w383, "XScale.Flipped"=FALSE ("X Scale.Flipped")) -> ()  [unwired: 2 in, 2 out]
          }
          frame #1 {
            w436 = 25000.0 ("rate")
            w438 = 10178 items=["Finite Samples"=10178, "Continuous Samples"=10123, "Hardware Timed Single Point"=12522] ("sample mode")
            w440 = 10178 items=["Finite Samples"=10178, "Continuous Samples"=10123, "Hardware Timed Single Point"=12522] ("sample mode")
            n271 = local read "Econtrol"() -> (w443:refnum<k21>)
            n272 = local read "Monitor"() -> (w441:refnum<k21>)
            n273 = call <vilib>:"DAQmx Stop Task.vi"("task/channels in"=w443) -> ("task out"=w442:refnum<k21>, "error out"=w444:errorcluster)  [unwired: 13 in]
            n274 = call-poly <vilib>:"DAQmx Timing.vi"("task/channels in"=w442, "sample mode"=w440, "samples per channel"=w427, "rate"=w428, "error in"=w444) -> ("task out"=w435:refnum<k21>, "error out"=w433:errorcluster)  [unwired: 9 in]
            n275 = Divide(x=w436, y=w428) -> (x/y=w430:dbl)
            n276 = Multiply(x=w430, y=w427) -> (x*y=w426:dbl)
            n277 = call-poly <vilib>:"DAQmx Timing.vi"("task/channels in"=w441, "sample mode"=w438, "samples per channel"=w426, "rate"=w436, "source"=tag "OnboardClock") -> ("task out"=w429:refnum<k21>)  [unwired: 9 in, 1 out]
            n278 = call-poly <vilib>:"DAQmx Trigger.vi"("task/channels in"=w435, "source"=tag "/cDAQ1/ai/StartTrigger", "error in"=w433) -> ("task out"=w432:refnum<k21>, "error out"=w431:errorcluster)  [unwired: 11 in]
            n279 = Two Button Dialog(message="Save CCD Data?", 1:"No" ("F button name (\"Cancel\")"), 2:"Yes" ("T button name (\"OK\")")) -> (T button?=w417:bool)
            n280 = case shown="False" w417 {
              tunnel: [path "" ("selected path") w446] -> w418
              frame False {
              }
              frame True {
                n281 = call "File Dialog2"() -> ("selected path"=w446:path)  [unwired: 12 in, 3 out]
              }
            }
            n282 = Multiply(x=w415, y=5.0) -> (x*y=w413:dbl[])
            n283 = local read "Cycle Time"() -> (w424:sgl)
            n284 = call-poly <vilib>:"DAQmx Write.vi"("task/channels in"=w432, "data"=w413, "error in"=w431) -> ("task out"=w439:refnum<k21>)  [unwired: 10 in, 2 out]
            n285 = Divide(x=w425, y=w424) -> (x/y=w423:dbl)
            n286 = Round Toward +Infinity(x=w423) -> (ceil(x): smallest int >= x=w422:dbl)
            n287 = To Long Integer(number=w422) -> (32bit integer=w416:i32)
            n288 = call <userlib>:"SetNumberKinetics.vi"("number"=w416) -> ()  [unwired: 1 in, 2 out]
          }
          frame #2 {
            w447 = dbl[] []
            n289 = local read "Binning"() -> (w452:i32)
            n290 = local read "xpixels"() -> (w454:i32)
            n291 = local read "ypixels"() -> (w453:i32)
            n292 = flat-sequence {
              tunnel: w473 -> [w534]
              tunnel: w472 -> [w535]
              tunnel: [w535] -> w469
              tunnel: [w533] -> w468
              tunnel: [w536] -> w471
              tunnel: [w537] -> w470
              tunnel: w469 -> [w538]
              tunnel: w468 -> [w536]
              frame #0 {
                n293 = call <vilib>:"DAQmx Start Task.vi"("task/channels in"=w534) -> ("task out"=w533:refnum<k21>)  [unwired: 13 in, 1 out]
              }
              frame #1 {
                n294 = call <vilib>:"DAQmx Start Task.vi"("task/channels in"=w538) -> ("task out"=w537:refnum<k21>)  [unwired: 13 in, 1 out]
              }
            }
            n295 = Divide(x=w454, y=w452) -> (x/y=w456:dbl)
            n296 = Divide(x=w453, y=w452) -> (x/y=w455:dbl)
            n297 = To Long Integer(number=w456) -> (32bit integer=w450:i32)
            n298 = To Long Integer(number=w455) -> (32bit integer=w449:i32)
            n299 = while {
              tunnel: w470 -> [w558]
              tunnel: w471 -> [_]
              tunnel: w467 -> [w539]
              shift-right: [w551] -> w464
              shift-left: w447 -> [w555]
              shift-right: [w541] -> w465
              shift-left: w447 -> [w544]
              tunnel: w466 -> [w553]
              stop <- w554 stop-if-true
              n300 = call-poly <vilib>:"DAQmx Read.vi"("task/channels in"=w558, "number of samples per channel"=w539) -> ("data"=w545:dbl[][])  [unwired: 11 in, 2 out]
              n301 = local read "Tip Gain (mV/pA)"() -> (w549:dbl)
              n302 = Index Array(array=w545, index (row)=0 ("index")) -> (element=w557:dbl[])  [unwired: 1 in]
              n303 = Index Array(array=w545, index (row)=1 ("index")) -> (element=w556:dbl[])  [unwired: 1 in]
              n304 = call-poly <vilib>:"Mean.vi"("X"=w557) -> ("mean"=w540:dbl)  [unwired: 1 out]
              n305 = call-poly <vilib>:"Mean.vi"("X"=w556) -> ("mean"=w543:dbl)  [unwired: 1 out]
              n306 = Multiply(x=w549, y=1000000000.0) -> (x*y=w546:dbl)
              n307 = Divide(x=w540, y=w546) -> (x/y=w547:dbl)
              n308 = Build Array (concatenate)(w544, w543) -> (w541:dbl[])
              n309 = Round Toward -Infinity(1:w553) -> (0:w552:dbl)
              n310 = Build Array (concatenate)(w555, w547) -> (w551:dbl[])
              n311 = Array Size(array=w541) -> (size(s)=w550:i32)
              "E-Chem Data Point" <- w550
              n312 = Greater Or Equal?(x=w550, y=w552) -> (x >= y?=w554:bool)
              n313 = Bundle(w541, w551) -> (→"Tip Voltammogram":cluster{dbl[], dbl[]})  [unwired: 1 in]
            }
            n314 = Multiply(x=w450, y=w449) -> (x*y=w451:i32)
            n315 = call <userlib>:"StartAcquisition.vi"() -> ("error out"=w458:errorcluster)  [unwired: 2 in, 1 out]
            n316 = local read "Background"() -> (w460:i32[][])
            n317 = while {
              tunnel: w462 -> [w493]
              tunnel: w461 -> [w492]
              tunnel: w460 -> [w491]
              shift-right: [w479] -> _
              shift-left: u32 0 ("y") -> [w488]
              tunnel: w458 -> [_]
              tunnel: w457 -> [w480]
              tunnel: w451 -> [w475]
              tunnel: w450 -> [w477]
              tunnel: w449 -> [w476]
              tunnel: w448 -> [w474]
              stop <- w483 stop-if-true
              w484 = 100.0 ("y")
              n318 = call <userlib>:"GetNumberNewImages.vi"() -> ("last"=w494:i32, "first"=w489:u32)  [unwired: 4 in, 2 out]
              n319 = Get Queue Status(queue=w474) -> (# elements in queue=w487:i32)  [unwired: 2 in, 7 out]
              n320 = Greater?(x=w489, y=w488) -> (0:w490:bool)
              n321 = Greater Than 0?(x=w487) -> (x > 0?=w486:bool)
              n322 = case shown="True" w490 {
                tunnel: w489 -> [_ w506]
                tunnel: w494 -> [_ w505]
                tunnel: w493 -> [_ w504]
                tunnel: w492 -> [_ w503]
                tunnel: [w497 w502] -> w479
                tunnel: w491 -> [_ w501]
                tunnel: w488 -> [w497 _]
                tunnel: w477 -> [_ w500]
                tunnel: w476 -> [_ w499]
                tunnel: w475 -> [_ w498]
                frame False {
                }
                frame True {
                  n323 = while {
                    tunnel: w505 -> [w512]
                    shift-right: [w517] -> _
                    shift-left: w506 -> [w514]
                    tunnel: w504 -> [w516]
                    tunnel: w503 -> [w515]
                    tunnel: [w512] -> w502
                    tunnel: w501 -> [w511]
                    tunnel: w500 -> [w510]
                    tunnel: w499 -> [w509]
                    tunnel: w498 -> [w508]
                    stop <- w513 stop-if-true
                    n324 = Initialize Array(0 ("element"), w508) -> (w522:i32[])
                    n325 = call <userlib>:"GetImages.vi"("first"=w514, "last"=w514, "array"=w522, "size"=w508) -> ("array"=w521:i32[])  [unwired: 7 in, 4 out]
                    n326 = Reverse 1D Array(array=w521) -> (reversed array=w520:i32[])
                    n327 = Reshape Array(w520, w509, w510) -> (w519:i32[][])
                    n328 = Transpose 2D Array(2D array=w519) -> (transposed array=w518:i32[][])
                    n329 = Subtract(x=w518, y=w511) -> (x-y=w507:i32[][])
                    n330 = case shown="True" w516 {
                      tunnel: w507 -> [_ w532]
                      tunnel: w515 -> [_ w526]
                      tunnel: w509 -> [_ w524]
                      frame False {
                      }
                      frame True {
                        n331 = local read "E-Chem Data Point"() -> (w525:i32)
                        n332 = Initialize Array(w525, w524) -> (w527:i32[])
                        n333 = Build Array (concatenate)(w527, w532) -> (w531:i32[][])
                        n334 = Transpose 2D Array(2D array=w531) -> (transposed array=w528:i32[][])
                        n335 = call-poly <vilib>:"Write Delimited Spreadsheet.vi"("file path (dialog if empty)"=w526, "2D data"=w528, "append to file? (new file:F)"=TRUE, "delimiter (\\t)"="," ("delimiter (\\t)")) -> ()  [unwired: 10 in, 2 out]
                      }
                    }
                    n336 = property on="CCD Image" class="IntGraph (strict)"("Value"=w507) -> ()  [unwired: 2 in, 2 out]
                    n337 = Greater Or Equal?(x=w514, y=w512) -> (x >= y?=w513:bool)
                    n338 = Increment(x=w514) -> (x+1=w517:u32)
                  }
                }
              }
              n339 = case shown="True" w486 {
                selector: w486 -> [w495 w496]
                tunnel: [w495 w496] -> w481
                frame False {
                }
                frame True {
                  n340 = call <userlib>:"AbortAcquisition.vi"() -> ()  [unwired: 2 in, 2 out]
                }
              }
              n341 = Divide(x=w479, y=w480) -> (x/y=w485:dbl)
              n342 = Multiply(x=w485, y=w484) -> (x*y=w478:dbl)
              n343 = Greater Or Equal?(x=w478, y=w484) -> (x >= y?=w482:bool)
              n344 = local write "Acquisition Progress"(w478) -> ()
              n345 = Or(x=w482, y=w481) -> (x .or. y?=w483:bool)
            }
            n346 = Build Array(w465, w464) -> (w463:dbl[][])
          }
          frame #3 {
            w569 = 10123 items=["Finite Samples"=10178, "Continuous Samples"=10123, "Hardware Timed Single Point"=12522] ("sample mode")
            n347 = Two Button Dialog(message="Save CV?", 1:"No" ("F button name (\"Cancel\")"), 2:"Yes" ("T button name (\"OK\")")) -> (T button?=w564:bool)
            n348 = Enqueue Element(queue=w573, element=SpectroElectroChem_1Electrode_caseEnum."Set E") -> (queue out=w562:refnum<queue>)  [unwired: 2 in, 2 out]
            n349 = case shown="True" w564 {
              tunnel: w563 -> [_ w577]
              frame False {
              }
              frame True {
                n350 = Transpose 2D Array(2D array=w577) -> (transposed array=w576:dbl[][])
                n351 = call-poly <vilib>:"Write Delimited Spreadsheet.vi"("format (%.3f)"="%.3e", "2D data"=w576) -> ()  [unwired: 12 in, 2 out]
              }
            }
            n352 = Enqueue Element(queue=w562, element=SpectroElectroChem_1Electrode_caseEnum."Setup CCD") -> ()  [unwired: 2 in, 3 out]
            n353 = call <vilib>:"DAQmx Stop Task.vi"("task/channels in"=w572) -> ("task out"=w571:refnum<k21>)  [unwired: 13 in, 1 out]
            n354 = call-poly <vilib>:"DAQmx Timing.vi"("task/channels in"=w571, "sample mode"=w569, "rate"=25000.0, "source"=tag "OnboardClock") -> ()  [unwired: 10 in, 2 out]
          }
        }
      }
      frame "Acquire SECCM Image" {
        n355 = stacked-sequence {
          seq-local: [_ w590 _ _ _ _ _ _] -> [_ _ _ _ _ _ _ _]
          seq-local: [_ w589 _ _ _ _ _ _] -> [_ _ _ _ _ _ _ _]
          seq-local: [_ w587 _ _ _ _ _ _] -> [_ _ _ w653 _ _ _ _]
          seq-local: [_ _ _ w633 _ _ _ _] -> [_ _ _ _ _ _ _ w996]
          seq-local: [_ _ w600 _ _ _ _ _] -> [_ _ _ w647 _ _ _ _]
          seq-local: [_ _ "CV v / mV/s" _ _ _ _ _] -> [_ _ _ w646 _ _ _ _]
          seq-local: [_ _ w598 _ _ _ _ _] -> [_ _ _ w645 _ _ _ _]
          seq-local: [_ w587 _ _ _ _ _ _] -> [_ _ _ w644 _ _ _ _]
          seq-local: [_ _ _ w634 _ _ _ _] -> [_ _ _ _ w919 _ _ _]
          seq-local: [_ _ _ w629 _ _ _ _] -> [_ _ _ _ _ _ _ w964]
          tunnel: w578 -> [_ _ _ _ _ _ _ w1001]
          frame #0 {
            n356 = property on="SECCM Image" class="IntGraph (strict)"("XScale.Multiplier"="xy Res. / um", "XScale.Offset"="xi / um", "YScale.Multiplier"="xy Res. / um", "YScale.Offset"="yi / um", "XScale.Minimum"="xi / um", "XScale.Maximum"="xf / um", "YScale.Minimum"="yi / um", "YScale.Maximum"="yf / um") -> ()  [unwired: 2 in, 2 out]
            n357 = property on="Height Image" class="IntGraph (strict)"("XScale.Multiplier"="xy Res. / um", "XScale.Offset"="xi / um", "YScale.Multiplier"="xy Res. / um", "YScale.Offset"="yi / um", "XScale.Minimum"="xi / um", "XScale.Maximum"="xf / um", "YScale.Minimum"="yi / um", "YScale.Maximum"="yf / um") -> ()  [unwired: 2 in, 2 out]
          }
          frame #1 {
            n358 = local read "xy Res. / um"() -> (w591:dbl)
            n359 = local read "xf / um"() -> (w597:dbl)
            n360 = local read "xi / um"() -> (w596:dbl)
            n361 = local read "yf / um"() -> (w595:dbl)
            n362 = local read "yi / um"() -> (w594:dbl)
            n363 = Subtract(x=w595, y=w594) -> (x-y=w592:dbl)
            n364 = Subtract(x=w597, y=w596) -> (x-y=w593:dbl)
            n365 = Divide(x=w593, y=w591) -> (x/y=w586:dbl)
            n366 = Divide(x=w592, y=w591) -> (x/y=w585:dbl)
            n367 = To Long Integer(number=w586) -> (32bit integer=w590:i32)
            n368 = To Long Integer(number=w585) -> (32bit integer=w589:i32)
            n369 = Initialize Array(0.0 ("element"), w590, w589) -> (w587:dbl[][])
          }
          frame #2 {
            w605 = 0.05 ("y")
            w623 = 2.0 ("y")
            n370 = Add(x="CV Ef / V", y="CV Ei / V") -> (x+y=w624:dbl)
            n371 = Subtract(x="CV Ef / V", y="CV Ei / V") -> (x-y=w620:dbl)
            n372 = Absolute Value(x=w620) -> (abs(x)=w619:dbl)
            n373 = Multiply(x=w619, y=1000.0) -> (x*y=w618:dbl)
            n374 = Multiply(x=w618, y=2.0) -> (x*y=w615:dbl)
            n375 = Divide(x="CV v / mV/s", y=w615) -> (x/y=w614:dbl)
            n376 = Divide(x=w624, y=w623) -> (x/y=w622:dbl)
            n377 = Divide(x=w620, y=w623) -> (x/y=w625:dbl)
            n378 = Divide(x="CV v / mV/s", y=w614) -> (x/y=w613:dbl)
            n379 = Multiply(x=w613, y="CV Cycles") -> (x*y=w598:dbl)
            n380 = Bundle("CV v / mV/s"="CV v / mV/s", w598) -> (w611:cluster{"CV v / mV/s":dbl, dbl})  [unwired: 1 in]
            n381 = call <vilib>:"Triangle Waveform.vi"("offset"=w622, "sampling info"=w611, "reset signal"=TRUE, "phase"=270.0, "amplitude"=w625, "frequency"=w614) -> ("signal out"=w610:waveform(dbl))  [unwired: 4 in, 1 out]
            n382 = Unbundle By Name(w610) -> ("Y"=w601:dbl[])
            n383 = Multiply(x=w601, y=5.0) -> (x*y=w600:dbl[])
            n384 = Max & Min(x="CV Ef / V", y="CV Ei / V") -> (max(x,y)=w606:dbl, min(x,y)=w607:dbl)
            n385 = Add(x=w606, y=w605) -> (x+y=w604:dbl)
            n386 = Subtract(x=w607, y=w605) -> (x-y=w603:dbl)
            n387 = property on="Tip Voltammogram 2" class="XYGraph (strict)"("XScale.Maximum"=w604, "XScale.Minimum"=w603) -> ()  [unwired: 2 in, 2 out]
          }
          frame #3 {
            n388 = local read "xy Res. / um"() -> (w635:dbl)
            n389 = local read "xf / um"() -> (w637:dbl)
            n390 = local read "Piezo Axes"() -> (w657:string[])
            n391 = local read "xi / um"() -> (w638:dbl)
            n392 = local read "yf / um"() -> (w641:dbl)
            n393 = local read "yi / um"() -> (w642:dbl)
            n394 = Index Array(array=w657, index=0) -> (element=w650:string)
            n395 = Index Array(array=w657, index=1) -> (element=w649:string)
            n396 = Index Array(array=w657, index=2) -> (element=w656:string)
            n397 = Build Array(w650) -> (w655:string[])
            n398 = Build Array(w649) -> (w654:string[])
            n399 = Build Array(w656) -> (w627:string[])
            n400 = Build Array(w650, w649) -> (w648:string[])
            n401 = Subtract(x=w637, y=w638) -> (x-y=w639:dbl)
            n402 = Subtract(x=w641, y=w642) -> (x-y=w643:dbl)
            n403 = Divide(x="z Res. / um", y="t / s/pt") -> (x/y=w634:dbl)
            n404 = Build Array(w634) -> (w628:dbl[])
            n405 = call "VEL.vi"("Axes to set"=w627, "Velocity values"=w628) -> ()  [unwired: 16 in, 2 out]
            n406 = Divide(x=w639, y=w635) -> (x/y=w636:dbl)
            n407 = Divide(x=w643, y=w635) -> (x/y=w640:dbl)
            n408 = while {
              tunnel: w655 -> [w692]
              tunnel: w654 -> [w687]
              tunnel: w627 -> [w691]
              shift-right: [w684] -> w633
              shift-left: w653 -> [w685]
              tunnel: w648 -> [w683]
              tunnel: w647 -> [w682]
              tunnel: w646 -> [w681]
              tunnel: w645 -> [w680]
              tunnel: w634 -> [w679]
              shift-right: [w677] -> _
              shift-left: w644 -> [w678]
              tunnel: w640 -> [w671]
              tunnel: w636 -> [w670]
              tunnel: w635 -> [w665]
              tunnel: [w664] -> w631
              shift-right: [w663] -> w630
              shift-left: dbl[][] [] -> [w662]
              tunnel: w628 -> [w661]
              i -> [w669]
              stop <- w674 stop-if-true
              n409 = local read "yi / um"() -> (w690:dbl)
              n410 = Increment(x=w669) -> (x+1=w672:i32)
              n411 = Quotient & Remainder(x=w669, y=2) -> (x-y*floor(x/y)=w667:i32)  [unwired: 1 out]
              n412 = Multiply(x=w665, y=w669) -> (x*y=w689:dbl)
              n413 = Add(x=w690, y=w689) -> (x+y=w686:dbl)
              n414 = Build Array(w686) -> (w688:dbl[])
              n415 = local write "Sample y"(w686) -> ()
              n416 = call "MOV.vi"("Axes to move"=w687, "Position values"=w688) -> ("error out"=w673:errorcluster)  [unwired: 17 in]
              n417 = Equal To 0?(x=w667) -> (x = 0?=w666:bool)
              n418 = Greater Or Equal?(x=w672, y=w671) -> (x >= y?=w675:bool)
              n419 = while {
                tunnel: w692 -> [w721]
                tunnel: w691 -> [w718]
                tunnel: w687 -> [_]
                tunnel: w669 -> [w716]
                shift-right: [w715] -> w684
                shift-left: w685 -> [w717]
                tunnel: w683 -> [w714]
                tunnel: w682 -> [w713]
                tunnel: w681 -> [w712]
                tunnel: w680 -> [w711]
                tunnel: w679 -> [w710]
                shift-right: [w708] -> w677
                shift-left: w678 -> [w709]
                tunnel: ["Stop SECM Image"] -> w676
                tunnel: w673 -> [_]
                tunnel: w670 -> [w699]
                tunnel: w666 -> [w702]
                tunnel: w665 -> [w698]
                tunnel: [w696] -> w664
                shift-right: [w695] -> w663
                shift-left: w662 -> [w694]
                tunnel: w661 -> [w693]
                i -> [w700]
                stop <- w706 stop-if-true
                n420 = local read "xi / um"() -> (w720:dbl)
                n421 = case shown="False" w702 {
                  tunnel: w700 -> [w724 w727]
                  tunnel: [w723 w727] -> w697
                  tunnel: w699 -> [w726 _]
                  frame False {
                    n422 = Decrement(x=w726) -> (x-1=w725:dbl)
                    n423 = Subtract(x=w725, y=w724) -> (x-y=w723:dbl)
                  }
                  frame True {
                  }
                }
                n424 = Increment(x=w700) -> (x+1=w703:i32)
                n425 = Multiply(x=w698, y=w697) -> (x*y=w701:dbl)
                n426 = Add(x=w720, y=w701) -> (x+y=w719:dbl)
                n427 = Build Array(w719) -> (w722:dbl[])
                n428 = call "MOV.vi"("Axes to move"=w721, "Position values"=w722) -> ("error out"=w705:errorcluster)  [unwired: 17 in]
                n429 = local write "Sample x"(w719) -> ()
                n430 = Greater Or Equal?(x=w703, y=w699) -> (x >= y?=w704:bool)
                n431 = stacked-sequence {
                  seq-local: [_ _ _ _ _ _ _ w836 _ _ _] -> [_ _ _ _ _ _ _ _ w873 _ _]
                  seq-local: [_ _ _ _ _ _ _ w832 _ _ _] -> [_ _ _ _ _ _ _ _ w872 _ _]
                  seq-local: [_ _ _ _ _ _ _ w835 _ _ _] -> [_ _ _ _ _ _ _ _ w869 _ _]
                  seq-local: [_ _ _ _ w761 _ _ _ _ _ _] -> [_ _ _ _ _ _ _ _ _ _ _]
                  seq-local: [_ _ _ w755 _ _ _ _ _ _ _] -> [_ _ _ _ w760 _ _ _ _ _ _]
                  seq-local: [_ _ _ _ _ _ _ _ _ w906 _] -> [_ _ _ _ _ _ _ _ _ _ w912]
                  tunnel: w718 -> [_ _ _ w757 w759 w810 _ _ _ w902 w916]
                  tunnel: w717 -> [_ _ _ _ _ w827 _ _ _ _ _]
                  tunnel: w716 -> [_ _ _ _ _ w812 _ _ w864 _ _]
                  tunnel: w697 -> [_ _ _ _ _ w813 _ _ w865 _ _]
                  tunnel: [_ _ _ _ _ w826 _ _ _ _ _] -> w715
                  tunnel: w714 -> [_ _ _ _ _ _ _ _ _ _ _]
                  tunnel: [_ _ _ _ _ _ _ w852 _ _ _] -> _
                  tunnel: w713 -> [_ _ _ _ _ _ _ w852 _ _ _]
                  tunnel: w712 -> [_ _ _ _ _ _ _ w839 _ _ _]
                  tunnel: w711 -> [_ _ _ _ _ _ _ w840 w867 _ _]
                  tunnel: w710 -> [_ _ _ _ _ _ _ _ _ w901 _]
                  tunnel: w709 -> [_ _ _ _ _ _ _ _ w866 _ _]
                  tunnel: [_ _ _ _ _ _ _ _ w860 _ _] -> w708
                  tunnel: w705 -> [_ _ _ _ _ _ _ _ _ _ _]
                  tunnel: w698 -> [w728 _ _ _ _ _ _ _ _ _ _]
                  tunnel: [_ _ _ _ _ _ _ _ w859 _ _] -> w696
                  tunnel: [_ _ _ _ _ _ _ _ w857 _ _] -> w695
                  tunnel: w694 -> [_ _ _ _ _ _ _ _ w856 _ _]
                  tunnel: w693 -> [_ _ _ _ _ _ _ _ _ _ _]
                  frame #0 {
                    # "v"
                    n432 = Divide(x=w728, y=100.0) -> (x/y=w731:dbl)
                    n433 = Multiply(x=w731, y=1000.0) -> (x*y=w729:dbl)
                    n434 = Wait (ms)(milliseconds to wait=w729) -> ()  [unwired: 1 out]
                  }
                  frame #1 {
                    w746 = 10123 items=["Finite Samples"=10178, "Continuous Samples"=10123, "Hardware Timed Single Point"=12522] ("sample mode")
                    n435 = local read "Monitor"() -> (w737:refnum<k21>)
                    n436 = local read "Econtrol"() -> (w745:refnum<k21>)
                    n437 = Multiply(x="E Approach / V", y=5.0) -> (x*y=w751:dbl)
                    n438 = Initialize Array(w751, 2 ("dimension size")) -> (w753:dbl[])
                    n439 = call <vilib>:"DAQmx Stop Task.vi"("task/channels in"=w737) -> ("task out"=w743:refnum<k21>, "error out"=w742:errorcluster)  [unwired: 13 in]
                    n440 = call-poly <vilib>:"DAQmx Timing.vi"("task/channels in"=w743, "sample mode"=w746, "rate"=25000.0, "error in"=w742) -> ("task out"=w735:refnum<k21>, "error out"=w736:errorcluster)  [unwired: 10 in]
                    n441 = property class="DAQmx Read"(reference=w735, error in=w736, "AutoStart"=FALSE) -> (error out=w733:errorcluster)  [unwired: 1 out]
                    n442 = call <vilib>:"DAQmx Stop Task.vi"("task/channels in"=w745, "error in"=w733) -> ("task out"=w752:refnum<k21>, "error out"=w748:errorcluster)  [unwired: 12 in]
                    n443 = call-poly <vilib>:"DAQmx Write.vi"("task/channels in"=w752, "data"=w753, "error in"=w748) -> ("task out"=w738:refnum<k21>, "error out"=w740:errorcluster)  [unwired: 10 in, 1 out]
                    n444 = call-poly <vilib>:"DAQmx Trigger.vi"("task/channels in"=w738, "error in"=w740) -> ("task out"=w741:refnum<k21>, "error out"=w739:errorcluster)  [unwired: 12 in]
                    n445 = call <vilib>:"DAQmx Start Task.vi"("task/channels in"=w741, "error in"=w739) -> ()  [unwired: 12 in, 2 out]
                  }
                  frame #2 {
                    n446 = Wait (ms)(milliseconds to wait=u32 50) -> ()  [unwired: 1 out]
                  }
                  frame #3 {
                    n447 = local read "Monitor"() -> (w756:refnum<k21>)
                    n448 = call <vilib>:"DAQmx Start Task.vi"("task/channels in"=w756) -> ("task out"=w755:refnum<k21>)  [unwired: 13 in, 1 out]
                    n449 = call "MOV.vi"("Axes to move"=w757, "Position values"=dbl[] [85.0]) -> ()  [unwired: 17 in, 1 out]
                  }
                  frame #4 {
                    w764 = dbl[] []
                    n450 = local read "z Res. / um"() -> (w762:dbl)
                    n451 = local read "Piezo z"() -> (w763:dbl)
                    n452 = while {
                      shift-right: [w787] -> _
                      shift-left: w764 -> [w790]
                      shift-right: [w788] -> _
                      shift-left: w764 -> [w789]
                      tunnel: w763 -> [w778]
                      tunnel: w762 -> [w780]
                      tunnel: [w769] -> w761
                      tunnel: w760 -> [w772]
                      tunnel: w759 -> [w770]
                      i -> [w773]
                      stop <- w774 stop-if-true
                      n453 = local read "t / s/pt"() -> (w765:dbl)
                      n454 = local read "Tip Gain (mV/pA)"() -> (w792:dbl)
                      n455 = Multiply(x=w765, y=1000.0) -> (x*y=w767:dbl)
                      n456 = Multiply(x=w780, y=w773) -> (x*y=w779:dbl)
                      n457 = call-poly <vilib>:"DAQmx Read.vi"("task/channels in"=w772, "number of samples per channel"=-1) -> ("data"=w793:dbl[][])  [unwired: 11 in, 2 out]
                      n458 = Wait (ms)(milliseconds to wait=w767) -> ()  [unwired: 1 out]
                      n459 = Add(x=w779, y=w778) -> (x+y=w769:dbl)
                      n460 = Multiply(x=w765, y=25000.0) -> ()  [unwired: 1 out]
                      n461 = Multiply(x=w792, y=1000000000.0) -> (x*y=w775:dbl)
                      n462 = Index Array(array=w793, index (row)=0) -> (element=w795:dbl[])  [unwired: 1 in]
                      n463 = call-poly <vilib>:"Mean.vi"("X"=w795) -> ("mean"=w794:dbl)  [unwired: 1 out]
                      n464 = Equal?(x="SECCM SP Dir", y=u16 0) -> (x = y?=w783:bool)
                      n465 = Divide(x=w794, y=w775) -> (x/y=w781:dbl)
                      n466 = Build Array (concatenate)(w789, w769) -> (w788:dbl[])
                      n467 = case shown="False" w783 {
                        tunnel: "Approach Set / A" -> [w800 w803]
                        tunnel: w781 -> [w801 w804]
                        tunnel: [w799 w802] -> w771
                        frame False {
                          n468 = Less?(x=w801, y=w800) -> (x < y?=w799:bool)
                        }
                        frame True {
                          n469 = Greater?(x=w804, y=w803) -> (0:w802:bool)
                        }
                      }
                      n470 = case shown="True" w771 {
                        tunnel: w770 -> [_ w798]
                        frame False {
                        }
                        frame True {
                          n471 = call "STP.vi"("Affected axes?"=w798) -> ()  [unwired: 18 in, 1 out]
                        }
                      }
                      n472 = local write "Sample z"(w769) -> ()
                      n473 = local write "Piezo z"(w769) -> ()
                      n474 = Greater Or Equal?(x=w769, y=80.0) -> (x >= y?=w777:bool)
                      n475 = Build Array (concatenate)(w790, w781) -> (w787:dbl[])
                      n476 = Bundle(w788, w787) -> (→"Tip Approach Curve 2":cluster{dbl[], dbl[]})  [unwired: 1 in]
                      n477 = Or(x=w771, y=w777) -> (x .or. y?=w774:bool)
                    }
                  }
                  frame #5 {
                    n478 = local read "Monitor"() -> (w808:refnum<k21>)
                    n479 = local read "CV Ei / V"() -> (w818:dbl)
                    n480 = call "POS?.vi"("Axes to query"=w810) -> ("Position"=w829:dbl[])  [unwired: 17 in, 1 out]
                    n481 = Multiply(x=w818, y=5.0) -> (x*y=w819:dbl)
                    n482 = local read "Econtrol"() -> (w820:refnum<k21>)
                    n483 = call-poly <vilib>:"DAQmx Read.vi"("task/channels in"=w808, "number of samples per channel"=-1) -> ("task out"=w807:refnum<k21>, "error out"=w805:errorcluster)  [unwired: 11 in, 1 out]
                    n484 = Index Array(array=w829, index=0) -> (element=w811:dbl)
                    n485 = Replace Array Subset(array=w827, new element=w811, index (row)=w813, index (col)=w812) -> (w826:dbl[][])
                    "Height Image" <- w826
                    n486 = Initialize Array(w819, 2 ("dimension size")) -> (w823:dbl[])
                    n487 = local write "Sample z"(w811) -> ()
                    n488 = call <vilib>:"DAQmx Stop Task.vi"("task/channels in"=w807, "error in"=w805) -> ("error out"=w809:errorcluster)  [unwired: 12 in, 1 out]
                    n489 = local write "Piezo z"(w811) -> ()
                    n490 = call <vilib>:"DAQmx Stop Task.vi"("task/channels in"=w820, "error in"=w809) -> ("task out"=w822:refnum<k21>, "error out"=w815:errorcluster)  [unwired: 12 in]
                    n491 = call "getMinMax.vi"("Array"=w826) -> ("Max"=w824:dbl, "Min"=w825:dbl)  [unwired: 1 in]
                    n492 = property on="Height Image" class="IntGraph (strict)"("ZScale.Maximum"=w824, "ZScale.Minimum"=w825) -> ()  [unwired: 2 in, 2 out]
                    n493 = call-poly <vilib>:"DAQmx Write.vi"("task/channels in"=w822, "data"=w823, "error in"=w815) -> ("task out"=w821:refnum<k21>, "error out"=w814:errorcluster)  [unwired: 10 in, 1 out]
                    n494 = call <vilib>:"DAQmx Start Task.vi"("task/channels in"=w821, "error in"=w814) -> ()  [unwired: 12 in, 2 out]
                  }
                  frame #6 {
                    n495 = Wait (ms)(milliseconds to wait=u32 20) -> ()  [unwired: 1 out]
                  }
                  frame #7 {
                    w838 = 25000.0 ("rate")
                    w843 = 10178 items=["Finite Samples"=10178, "Continuous Samples"=10123, "Hardware Timed Single Point"=12522] ("sample mode")
                    w844 = 10178 items=["Finite Samples"=10178, "Continuous Samples"=10123, "Hardware Timed Single Point"=12522] ("sample mode")
                    n496 = local read "Econtrol"() -> (w848:refnum<k21>)
                    n497 = local read "Monitor"() -> (w841:refnum<k21>)
                    n498 = call <vilib>:"DAQmx Stop Task.vi"("task/channels in"=w848) -> ("task out"=w847:refnum<k21>, "error out"=w850:errorcluster)  [unwired: 13 in]
                    n499 = Divide(x=w838, y=w839) -> (x/y=w835:dbl)
                    n500 = Multiply(x=w840, y=w835) -> (x*y=w837:dbl)
                    n501 = call-poly <vilib>:"DAQmx Timing.vi"("task/channels in"=w847, "sample mode"=w844, "samples per channel"=w840, "rate"=w839, "error in"=w850) -> ("task out"=w846:refnum<k21>, "error out"=w849:errorcluster)  [unwired: 9 in]
                    n502 = call-poly <vilib>:"DAQmx Timing.vi"("task/channels in"=w841, "sample mode"=w843, "samples per channel"=w837, "rate"=w838, "source"=tag "OnboardClock") -> ("task out"=w833:refnum<k21>)  [unwired: 9 in, 1 out]
                    n503 = call-poly <vilib>:"DAQmx Trigger.vi"("task/channels in"=w846, "source"=tag "/cDAQ1/ai/StartTrigger", "error in"=w849) -> ("task out"=w845:refnum<k21>, "error out"=w851:errorcluster)  [unwired: 11 in]
                    n504 = property class="DAQmx Read"(reference=w833, "AutoStart"=TRUE) -> (reference out=w832:refnum<k21>)  [unwired: 1 in, 1 out]
                    n505 = call-poly <vilib>:"DAQmx Write.vi"("task/channels in"=w845, "data"=w852, "error in"=w851) -> ("task out"=w836:refnum<k21>)  [unwired: 10 in, 2 out]
                  }
                  frame #8 {
                    w868 = dbl[] []
                    n506 = flat-sequence {
                      tunnel: w873 -> [w897]
                      tunnel: w872 -> [w895]
                      tunnel: [w896] -> w871
                      tunnel: [w895] -> w870
                      tunnel: w871 -> [w899]
                      tunnel: w870 -> [w900]
                      tunnel: [w898] -> w855
                      frame #0 {
                        n507 = call <vilib>:"DAQmx Start Task.vi"("task/channels in"=w897) -> ("error out"=w896:errorcluster)  [unwired: 13 in, 1 out]
                      }
                      frame #1 {
                        n508 = call <vilib>:"DAQmx Start Task.vi"("task/channels in"=w900, "error in"=w899) -> ("task out"=w898:refnum<k21>)  [unwired: 12 in, 1 out]
                      }
                    }
                    n509 = call-poly <vilib>:"DAQmx Read.vi"("task/channels in"=w855, "number of samples per channel"=0) -> ("task out"=w853:refnum<k21>)  [unwired: 11 in, 2 out]
                    n510 = while {
                      tunnel: w853 -> [w878]
                      tunnel: w869 -> [w894]
                      shift-right: [w876] -> w858
                      shift-left: w868 -> [w881]
                      shift-right: [w880] -> w859
                      shift-left: w868 -> [w882]
                      tunnel: w867 -> [w874]
                      stop <- w877 stop-if-true
                      n511 = local read "Tip Gain (mV/pA)"() -> (w886:dbl)
                      n512 = call-poly <vilib>:"DAQmx Read.vi"("task/channels in"=w878, "number of samples per channel"=w894) -> ("data"=w893:dbl[][])  [unwired: 11 in, 2 out]
                      n513 = Multiply(x=w886, y=1000000000.0) -> (x*y=w887:dbl)
                      n514 = Index Array(array=w893, index (row)=1) -> (element=w889:dbl[])  [unwired: 1 in]
                      n515 = Index Array(array=w893, index (row)=0) -> (element=w890:dbl[])  [unwired: 1 in]
                      n516 = call-poly <vilib>:"Mean.vi"("X"=w889) -> ("mean"=w883:dbl)  [unwired: 1 out]
                      n517 = Build Array (concatenate)(w882, w883) -> (w880:dbl[])
                      n518 = call-poly <vilib>:"Mean.vi"("X"=w890) -> ("mean"=w885:dbl)  [unwired: 1 out]
                      n519 = Divide(x=w885, y=w887) -> (x/y=w884:dbl)
                      n520 = Build Array (concatenate)(w881, w884) -> (w876:dbl[])
                      n521 = Bundle(w880, w876) -> (→"Tip Voltammogram 2":cluster{dbl[], dbl[]})  [unwired: 1 in]
                      n522 = Array Size(array=w876) -> (size(s)=w875:i32)
                      n523 = Greater Or Equal?(x=w875, y=w874) -> (x >= y?=w877:bool)
                    }
                    n524 = call-poly <vilib>:"Mean.vi"("X"=w858) -> ("mean"=w863:dbl)  [unwired: 1 out]
                    n525 = Replace Array Subset(array=w866, new element=w863, index (row)=w865, index (col)=w864) -> (w860:dbl[][])
                    "SECM Image" <- w860
                    n526 = call "getMinMax.vi"("Array"=w860) -> ("Max"=w861:dbl, "Min"=w862:dbl)  [unwired: 1 in]
                    n527 = property on="SECCM Image" class="IntGraph (strict)"("ZScale.Maximum"=w861, "ZScale.Minimum"=w862) -> ()  [unwired: 2 in, 2 out]
                    n528 = Build Array (concatenate)(w856, w858) -> (w857:dbl[][])
                  }
                  frame #9 {
                    (unwired) dbl[] [100.0] ("Velocity values")
                    n529 = local read "Piezo z"() -> (w909:dbl)
                    n530 = Subtract(x=w909, y="Retraction / um") -> (x-y=w910:dbl)
                    n531 = Divide(x="Retraction / um", y=w901) -> (x/y=w905:dbl)
                    n532 = Add(x=w905, y=0.05) -> (x+y=w904:dbl)
                    n533 = Build Array(w910) -> (w911:dbl[])
                    n534 = call "MOV.vi"("Axes to move"=w902, "Position values"=w911) -> ("error out"=w908:errorcluster)  [unwired: 17 in]
                    n535 = call "Time Delay2"("error in (no error)"=w908, "Delay Time (s)"=w904) -> ("error out"=w906:errorcluster)  [unwired: 9 in]
                  }
                  frame #10 {
                    n536 = call "POS?.vi"("Axes to query"=w916, "error in"=w912) -> ("Position"=w915:dbl[])  [unwired: 16 in, 1 out]
                    n537 = Index Array(array=w915, index=0) -> (element=w913:dbl)
                    n538 = local write "Sample z"(w913) -> ()
                    n539 = local write "Piezo z"(w913) -> ()
                  }
                }
                n540 = Or(x="Stop SECM Image", y=w704) -> (x .or. y?=w706:bool)
              }
              n541 = Or(x=w676, y=w675) -> (x .or. y?=w674:bool)
            }
            n542 = Build Array (concatenate)(w631, w630) -> (w629:dbl[][])
          }
          frame #4 {
            n543 = flat-sequence {
              tunnel: w919 -> [w930]
              tunnel: [w927] -> w918
              tunnel: [w926] -> w917
              tunnel: w918 -> [w939]
              tunnel: w917 -> [_]
              frame #0 {
                n544 = local read "Piezo Axes"() -> (w937:string[])
                n545 = Index Array(array=w937, index=2) -> (element=w938:string)
                n546 = Build Array(w938) -> (w934:string[])
                n547 = call "POS?.vi"("Axes to query"=w934) -> ("Position"=w932:dbl[], "error out"=w933:errorcluster)  [unwired: 17 in]
                n548 = Index Array(array=w932, index=0) -> (element=w921:dbl)
                n549 = Subtract(x=w921, y=5.0) -> (x-y=w924:dbl)
                n550 = Max & Min(x=w924, y=0.0) -> (max(x,y)=w920:dbl)  [unwired: 1 out]
                n551 = Subtract(x=w921, y=w920) -> (x-y=w922:dbl)
                n552 = Divide(x=w922, y=w930) -> (x/y=w929:dbl)
                n553 = Multiply(x=w929, y=1000.0) -> (x*y=w927:dbl)
                n554 = Build Array(w920) -> (w935:dbl[])
                n555 = local write "Sample z"(w920) -> ()
                n556 = call "MOV.vi"("Axes to move"=w934, "Position values"=w935, "error in"=w933) -> ("error out"=w926:errorcluster)  [unwired: 16 in]
              }
              frame #1 {
                n557 = Wait (ms)(milliseconds to wait=w939) -> ()  [unwired: 1 out]
              }
            }
          }
          frame #5 {
            n558 = local read "Piezo Axes"() -> (w945:string[])
            n559 = local read "xi / um"() -> (w942:dbl)
            n560 = local read "yi / um"() -> (w940:dbl)
            n561 = Index Array(array=w945, index=0) -> (element=w946:string)
            n562 = Index Array(array=w945, index=1) -> (element=w941:string)
            n563 = Build Array(w946, w941) -> (w944:string[])
            n564 = local write "Sample y"(w940) -> ()
            n565 = local write "Sample x"(w942) -> ()
            n566 = Build Array(w942, w940) -> (w943:dbl[])
            n567 = call "MOV.vi"("Axes to move"=w944, "Position values"=w943) -> ()  [unwired: 17 in, 1 out]
          }
          frame #6 {
            # "v"
            n568 = local read "xf / um"() -> (w956:dbl)
            n569 = local read "yf / um"() -> (w954:dbl)
            n570 = local read "yi / um"() -> (w953:dbl)
            n571 = local read "xi / um"() -> (w955:dbl)
            n572 = Subtract(x=w956, y=w955) -> (x-y=w952:dbl)
            n573 = Subtract(x=w954, y=w953) -> (x-y=w951:dbl)
            n574 = Add(x=w952, y=w951) -> (x+y=w950:dbl)
            n575 = Divide(x=w950, y=100.0) -> (x/y=w958:dbl)
            n576 = Multiply(x=w958, y=1000.0) -> (x*y=w949:dbl)
            n577 = Wait (ms)(milliseconds to wait=w949) -> ()  [unwired: 1 out]
          }
          frame #7 {
            w978 = T3 0 items=["no dialog", "OK message", "continue or stop message", "OK message + warnings", "continue/stop + warnings"] ("type of dialog (OK msg:1)")
            w980 = dbl[] [100.0, 100.0, 100.0] ("Velocity values")
            w992 = 10123 items=["Finite Samples"=10178, "Continuous Samples"=10123, "Hardware Timed Single Point"=12522] ("sample mode")
            n578 = local read "Piezo Axes"() -> (w981:string[])
            n579 = call "POS?.vi"("Axes to query"=w981) -> ("Position"=w989:dbl[], "error out"=w982:errorcluster)  [unwired: 17 in]
            n580 = Enqueue Element(queue=w1001, element=SpectroElectroChem_1Electrode_caseEnum."Rest") -> ()  [unwired: 2 in, 3 out]
            n581 = Index Array(array=w989, index=1) -> (element=w984:dbl)
            n582 = Index Array(array=w989, index=0) -> (element=w985:dbl)
            n583 = Index Array(array=w989, index=2) -> (element=w983:dbl)
            n584 = local write "Piezo x"(w985) -> ()
            n585 = local write "Piezo y"(w984) -> ()
            n586 = local write "Piezo z"(w983) -> ()
            n587 = Two Button Dialog(message="Save Height Image?", 1:"No" ("F button name (\"Cancel\")"), 2:"Yes" ("T button name (\"OK\")")) -> (T button?=w997:bool)
            n588 = call "VEL.vi"("Axes to set"=w981, "Velocity values"=w980, "error in"=w982) -> ("error out"=w979:errorcluster)  [unwired: 15 in, 1 out]
            n589 = Two Button Dialog(message="Save CV Data?", 1:"No" ("F button name (\"Cancel\")"), 2:"Yes" ("T button name (\"OK\")")) -> (T button?=w961:bool)
            n590 = local read "WE Rest E (V)"() -> (w965:dbl)
            n591 = local write "Piezo Velocity / um/s"(w980) -> ()
            n592 = case shown="True" w997 {
              tunnel: w996 -> [_ w1007]
              frame False {
              }
              frame True {
                n593 = Transpose 2D Array(2D array=w1007) -> (transposed array=w1006:dbl[][])
                n594 = call-poly <vilib>:"Write Delimited Spreadsheet.vi"("format (%.3f)"="%.6e", "2D data"=w1006) -> ()  [unwired: 12 in, 2 out]
              }
            }
            n595 = case shown="True" w961 {
              tunnel: w964 -> [_ w1004]
              frame False {
              }
              frame True {
                n596 = Transpose 2D Array(2D array=w1004) -> (transposed array=w1003:dbl[][])
                n597 = call-poly <vilib>:"Write Delimited Spreadsheet.vi"("format (%.3f)"="%.3e", "2D data"=w1003) -> ()  [unwired: 12 in, 2 out]
              }
            }
            n598 = Multiply(x=w965, y=5.0) -> (x*y=w975:dbl)
            n599 = local read "Econtrol"() -> (w971:refnum<k21>)
            n600 = Initialize Array(w975, 2 ("dimension size")) -> (w977:dbl[])
            n601 = call <vilib>:"DAQmx Stop Task.vi"("task/channels in"=w971) -> ("task out"=w976:refnum<k21>, "error out"=w972:errorcluster)  [unwired: 13 in]
            n602 = call <vilib>:"Simple Error Handler.vi"("type of dialog (OK msg:1)"=w978, "error in (no error)"=w979) -> ()  [unwired: 3 in, 5 out]
            n603 = call-poly <vilib>:"DAQmx Write.vi"("task/channels in"=w976, "data"=w977, "error in"=w972) -> ("task out"=w970:refnum<k21>, "error out"=w969:errorcluster)  [unwired: 10 in, 1 out]
            n604 = local read "Monitor"() -> (w990:refnum<k21>)
            n605 = call-poly <vilib>:"DAQmx Trigger.vi"("task/channels in"=w970, "error in"=w969) -> ("task out"=w967:refnum<k21>, "error out"=w968:errorcluster)  [unwired: 12 in]
            n606 = call <vilib>:"DAQmx Stop Task.vi"("task/channels in"=w990) -> ("task out"=w994:refnum<k21>)  [unwired: 13 in, 1 out]
            n607 = call <vilib>:"DAQmx Start Task.vi"("task/channels in"=w967, "error in"=w968) -> ("error out"=w966:errorcluster)  [unwired: 12 in, 1 out]
            n608 = call-poly <vilib>:"DAQmx Timing.vi"("task/channels in"=w994, "sample mode"=w992, "rate"=25000.0, "source"=tag "OnboardClock", "error in"=w966) -> ()  [unwired: 9 in, 2 out]
          }
        }
      }
      frame "Change Grating" {
        n609 = local read "Grating"() -> (w1009:u16)
        n610 = Increment(x=w1009) -> (x+1=w1008:u16)
        n611 = stacked-sequence {
          tunnel: w1010 -> [_ _ _ _ w1031]
          tunnel: w1008 -> [w1012 _ w1021 _ _]
          frame #0 {
            w1016 = FALSE ("SetTurret")
            n612 = call "shamrock_gratingsAction.vi"("WavelengthReset"=FALSE, 7:"Grating"=w1012, 8:"Grating"=w1012, "SetGrating"=TRUE, "SetGratingOffset"=FALSE, "SetTurret"=w1016, "Device No"=0, "SetDetectorOffset"=w1016) -> ()  [unwired: 3 in, 5 out]
          }
          frame #1 {
            n613 = call "shamrock_gratings.vi"("Device No"=0) -> ("lines/mm"=w1018:dbl)  [unwired: 1 in, 17 out]
            n614 = local write "Lines/mm"(w1018) -> ()
          }
          frame #2 {
            n615 = call "shamrock_wavelength.vi"("Grating No"=w1021, "Device No"=0) -> ("Wavelength"=w1020:dbl)  [unwired: 8 out]
            n616 = local write "Center Wavelength (nm)"(w1020) -> ()
            n617 = local write "Center"(w1020) -> ()
          }
          frame #3 {
            n618 = call "shamrock_calibrationAction.vi"("Device No"=0, "Set Pixel Width"=sgl 16.0, "Set Number Pixels"=1600) -> ("Wavelength First Pixel"=w1027:sgl, "Wavelength Last Pixel"=w1026:sgl)  [unwired: 3 out]
            n619 = local read "Binning"() -> (w1025:i32)
            n620 = local read "Center"() -> (w1024:dbl)
            n621 = control-ref of="CCD Image"() -> (w1023:refnum<vi>)
            n622 = local write "Right"(w1026) -> ()
            n623 = local write "Left"(w1027) -> ()
            n624 = call "configGraphX.vi"("Graph"=w1023, "min"=w1027, "max"=w1026, "Center"=w1024, "Binning"=w1025) -> ()  [unwired: 11 in]
          }
          frame #4 {
            n625 = Enqueue Element(queue=w1031, element=SpectroElectroChem_1Electrode_caseEnum."Clear CCD BG") -> ()  [unwired: 2 in, 3 out]
          }
        }
      }
      frame "Move Grating" {
        n626 = local read "Center Wavelength (nm)"() -> (w1036:dbl)
        n627 = local read "Grating"() -> (w1035:u16)
        n628 = Increment(x=w1035) -> (x+1=w1034:u16)
        n629 = stacked-sequence {
          tunnel: w1036 -> [w1038 _ _ _]
          tunnel: w1034 -> [_ w1043 _ _]
          tunnel: w1033 -> [_ _ _ w1054]
          frame #0 {
            n630 = call "shamrock_wavelengthAction.vi"("GoToZeroOrder"=FALSE, "Wavelength"=w1038, "SetWavelength"=TRUE, "Device No"=0) -> ()  [unwired: 2 out]
          }
          frame #1 {
            n631 = call "shamrock_wavelength.vi"("Grating No"=w1043, "Device No"=0) -> ("Wavelength"=w1042:dbl)  [unwired: 8 out]
            n632 = local write "Center Wavelength (nm)"(w1042) -> ()
            n633 = local write "Center"(w1042) -> ()
          }
          frame #2 {
            n634 = local read "Binning"() -> (w1046:i32)
            n635 = call "shamrock_calibrationAction.vi"("Device No"=0, "Set Pixel Width"=sgl 16.0, "Set Number Pixels"=1600) -> ("Wavelength First Pixel"=w1049:sgl, "Wavelength Last Pixel"=w1048:sgl)  [unwired: 3 out]
            n636 = local read "Center"() -> (w1047:dbl)
            n637 = control-ref of="CCD Image"() -> (w1045:refnum<vi>)
            n638 = local write "Left"(w1049) -> ()
            n639 = local write "Right"(w1048) -> ()
            n640 = call "configGraphX.vi"("Graph"=w1045, "min"=w1049, "max"=w1048, "Center"=w1047, "Binning"=w1046) -> ()  [unwired: 11 in]
          }
          frame #3 {
            n641 = Enqueue Element(queue=w1054, element=SpectroElectroChem_1Electrode_caseEnum."Clear CCD BG") -> ()  [unwired: 2 in, 3 out]
          }
        }
      }
      frame "Adjust Slit" {
        w1059 = 0.0 ("x")
        w1061 = 2400.0 ("y")
        n642 = local read "Slit Width (um)"() -> (w1057:dbl)
        n643 = Greater?(x=w1057, y=w1061) -> (0:w1062:bool)
        n644 = case shown="False" w1062 {
          tunnel: w1057 -> [w1076 _]
          tunnel: w1061 -> [_ w1077]
          tunnel: [w1076 w1077] -> w1058
          frame False {
          }
          frame True {
          }
        }
        n645 = Greater?(x=w1059, y=w1058) -> (0:w1060:bool)
        n646 = case shown="True" w1060 {
          tunnel: w1059 -> [_ w1075]
          tunnel: [w1074 w1075] -> w1056
          tunnel: w1058 -> [w1074 _]
          frame False {
          }
          frame True {
          }
        }
        n647 = stacked-sequence {
          tunnel: w1056 -> [w1064 _ _]
          tunnel: w1055 -> [_ _ w1073]
          frame #0 {
            n648 = call "shamrock_ioSlitAction.vi"("SetSlit"=TRUE, "Slit Width"=w1064, "Device No"=0, "SetOuputSlit"=FALSE, "Reset Slit"=FALSE, "Reset Output Slit"=FALSE) -> ()  [unwired: 1 in, 4 out]
          }
          frame #1 {
            n649 = call "shamrock_ioSlit.vi"("Device No"=0) -> ("Slit width (mm)"=w1070:dbl)  [unwired: 7 out]
            n650 = local write "Slit Width (um)"(w1070) -> ()
          }
          frame #2 {
            n651 = Enqueue Element(queue=w1073, element=SpectroElectroChem_1Electrode_caseEnum."Clear CCD BG") -> ()  [unwired: 2 in, 3 out]
          }
        }
      }
      frame "Setup CCD" {
        w1097 = sgl 0.0 ("Acc. Cycle Time")
        n652 = local read "Exp. Time"() -> (w1090:sgl)
        n653 = local read "# of Acc."() -> (w1089:i32)
        n654 = local read "EM Gain"() -> (w1091:i32)
        n655 = local read "ypixels"() -> (w1092:i32)
        n656 = local read "Binning"() -> (w1082:i32)
        n657 = local read "xpixels"() -> (w1093:i32)
        n658 = local read "HSS (MHz)"() -> (w1095:i32)
        n659 = local read "VSS (us)"() -> (w1094:i32)
        n660 = Enqueue Element(queue=w1079, element=SpectroElectroChem_1Electrode_caseEnum."Clear CCD BG") -> ()  [unwired: 2 in, 3 out]
        n661 = call "configKinMode.vi"("X Pixels"=w1093, "Y Pixels"=w1092, "Binning"=w1082, "EM Gain"=w1091, "Exp. Time"=w1090, "Acc. Cycle Time"=w1097, "Kin. Cycle Time"=w1097, "# of Acc."=w1089, "HSS"=w1095, "# of Scans"=1, "VSS"=w1094) -> ("Actual Kin. Cycle Time"=w1088:sgl)  [unwired: 13 in, 3 out]
        n662 = local write "Cycle Time"(w1088) -> ()
        n663 = control-ref of="CCD Image"() -> (w1087:refnum<vi>)
        n664 = local read "Right"() -> (w1085:dbl)
        n665 = local read "Center"() -> (w1086:dbl)
        n666 = local read "Left"() -> (w1084:dbl)
        n667 = call "configGraphX.vi"("Graph"=w1087, "min"=w1084, "max"=w1085, "Center"=w1086, "Binning"=w1082) -> ()  [unwired: 11 in]
        n668 = Multiply(x=0.16, y=w1082) -> (x*y=w1080:dbl)
        n669 = property on="CCD Image" class="IntGraph (strict)"("YScale.Multiplier"=w1080, "YScale.Maximum"=32.0 ("Y Scale.Range:Maximum")) -> ()  [unwired: 2 in, 2 out]
        n670 = property on="Total Intensity" class="IntGraph (strict)"("XScale.Multiplier"=w1080) -> ()  [unwired: 2 in, 2 out]
      }
      frame "Acquire CCD BG" {
        n671 = local read "Binning"() -> (w1106:i32)
        n672 = local read "xpixels"() -> (w1104:i32)
        n673 = local read "ypixels"() -> (w1105:i32)
        n674 = local read "Cycle Time"() -> (w1115:sgl)
        n675 = Divide(x=w1104, y=w1106) -> (x/y=w1112:dbl)
        n676 = Divide(x=w1105, y=w1106) -> (x/y=w1113:dbl)
        n677 = To Long Integer(number=w1112) -> (32bit integer=w1108:i32)
        n678 = To Long Integer(number=w1113) -> (32bit integer=w1107:i32)
        n679 = Multiply(x=w1115, y=sgl 10.0) -> (x*y=w1116:sgl)
        n680 = Multiply(x=w1108, y=w1107) -> (x*y=w1114:i32)
        n681 = To Unsigned Long Integer(number=w1114) -> (unsigned 32bit integer=w1109:u32)
        n682 = Initialize Array(0.0 ("element"), w1108, w1107) -> (w1110:dbl[][])
        n683 = while {
          shift-right: [w1126] -> w1099
          shift-left: w1110 -> [w1127]
          tunnel: w1116 -> [w1124]
          tunnel: w1109 -> [w1123]
          tunnel: w1108 -> [w1122]
          tunnel: w1107 -> [w1121]
          tunnel: w1103 -> [w1120]
          tunnel: [w1119] -> w1102
          i -> [w1125]
          stop <- w1129 stop-if-true
          n684 = call <userlib>:"StartAcquisition.vi"() -> ("error out"=w1138:errorcluster)  [unwired: 2 in, 1 out]
          n685 = while {
            tunnel: w1138 -> [_]
            tunnel: w1121 -> [w1145]
            tunnel: w1122 -> [w1144]
            tunnel: w1123 -> [w1143]
            tunnel: w1124 -> [w1142]
            tunnel: w1127 -> [w1141]
            tunnel: w1125 -> [w1140]
            tunnel: [w1139] -> w1126
            stop <- w1146 stop-if-true
            n686 = call <userlib>:"GetNumberAvailableImages.vi"() -> ("first"=w1149:i32)  [unwired: 3 in, 3 out]
            n687 = Wait (ms)(milliseconds to wait=w1142) -> ()  [unwired: 1 out]
            n688 = Greater Or Equal?(x=w1149, y=1) -> (x >= y?=w1147:bool)
            n689 = case shown="True" w1147 {
              selector: w1147 -> [w1151 w1167]
              tunnel: [w1151 w1167] -> w1146
              tunnel: w1145 -> [_ w1163]
              tunnel: w1144 -> [_ w1162]
              tunnel: w1143 -> [_ w1161]
              tunnel: w1141 -> [w1150 w1158]
              tunnel: w1140 -> [_ w1154]
              tunnel: [w1150 w1152] -> w1139
              frame False {
              }
              frame True {
                n690 = Multiply(x=w1158, y=w1154) -> (x*y=w1157:dbl[][])
                n691 = Increment(x=w1154) -> (x+1=w1153:i32)
                n692 = Initialize Array(0 ("element"), w1161) -> (w1165:i32[])
                n693 = call <userlib>:"GetMostRecentImage.vi"("size"=w1161, "array"=w1165) -> ("array"=w1160:i32[])  [unwired: 1 in, 2 out]
                n694 = Reverse 1D Array(array=w1160) -> (reversed array=w1164:i32[])
                n695 = Reshape Array(w1164, w1163, w1162) -> (w1159:i32[][])
                n696 = Transpose 2D Array(2D array=w1159) -> (transposed array=w1156:i32[][])
                n697 = Add(x=w1156, y=w1157) -> (x+y=w1155:dbl[][])
                n698 = Divide(x=w1155, y=w1153) -> (x/y=w1152:dbl[][])
                n699 = local write "CCD Image"(w1152) -> ()
              }
            }
          }
          n700 = Increment(x=w1125) -> (x+1=w1131:i32)
          n701 = Divide(x=w1131, y="Background \nFrames") -> (x/y=w1133:dbl)
          n702 = Multiply(x=w1133, y=100.0) -> (x*y=→"Acquisition Progress":dbl)
          n703 = Get Queue Status(queue=w1120) -> (queue out=w1119:refnum<queue>, # elements in queue=w1136:i32)  [unwired: 2 in, 6 out]
          n704 = Greater Than 0?(x=w1136) -> (x > 0?=w1137:bool)
          n705 = Increment(x=w1125) -> (x+1=w1134:i32)
          n706 = Greater Or Equal?(x=w1134, y="Background \nFrames") -> (x >= y?=w1135:bool)
          n707 = Or(x=w1135, y=w1137) -> (x .or. y?=w1129:bool)
        }
        n708 = To Long Integer(number=w1099) -> (32bit integer=w1100:i32[][])
        n709 = local write "Background"(w1100) -> ()
        n710 = Enqueue Element(queue=w1102, element=SpectroElectroChem_1Electrode_caseEnum."Rest") -> ()  [unwired: 2 in, 3 out]
      }
      frame "Clear CCD BG" {
        n711 = local read "ypixels"() -> (w1172:i32)
        n712 = local read "xpixels"() -> (w1171:i32)
        n713 = local read "Binning"() -> (w1173:i32)
        n714 = Enqueue Element(queue=w1169, element=SpectroElectroChem_1Electrode_caseEnum."Rest") -> ()  [unwired: 2 in, 3 out]
        n715 = Divide(x=w1171, y=w1173) -> (x/y=w1177:dbl)
        n716 = Divide(x=w1172, y=w1173) -> (x/y=w1178:dbl)
        n717 = To Long Integer(number=w1177) -> (32bit integer=w1176:i32)
        n718 = To Long Integer(number=w1178) -> (32bit integer=w1175:i32)
        n719 = Initialize Array(0.0 ("element"), w1176, w1175) -> (w1170:dbl[][])
        n720 = local write "Background"(w1170) -> ()
      }
      frame "Move Stage" {
      }
      frame "Acquire HSI" {
        n721 = local read "Binning"() -> (w1199:i32)
        n722 = local read "ypixels"() -> (w1200:i32)
        n723 = local read "xpixels"() -> (w1201:i32)
        n724 = Two Button Dialog(message="Save data?", 1:"No" ("F button name (\"Cancel\")"), 2:"Yes" ("T button name (\"OK\")")) -> (T button?=w1186:bool)
        n725 = Divide(x=w1201, y=w1199) -> (x/y=w1203:dbl)
        n726 = Divide(x=w1200, y=w1199) -> (x/y=w1202:dbl)
        n727 = Subtract(x="Final x (um)", y="Initial x (um)") -> (x-y=w1197:dbl)
        n728 = To Long Integer(number=w1203) -> (32bit integer=w1184:i32)
        n729 = To Long Integer(number=w1202) -> (32bit integer=w1182:i32)
        n730 = property on="Total Intensity" class="IntGraph (strict)"("YScale.Multiplier"="x Step (um)", "YScale.Offset"="Initial x (um)") -> ()  [unwired: 2 in, 2 out]
        n731 = case shown="True" w1186 {
          tunnel: [path "" ("selected path") w1213] -> w1185
          frame False {
          }
          frame True {
            n732 = call "File Dialog"() -> ("selected path"=w1213:path)  [unwired: 12 in, 3 out]
          }
        }
        n733 = Divide(x=w1197, y="x Step (um)") -> (x/y=w1196:dbl)
        n734 = Increment(x=w1196) -> (x+1=w1195:dbl)
        n735 = Multiply(x=w1184, y=w1182) -> (x*y=w1183:i32)
        n736 = Round Toward -Infinity(1:w1195) -> (0:w1181:dbl)
        n737 = Initialize Array(0.0 ("element"), w1182, w1181) -> (w1191:dbl[][])
        n738 = local read "Cycle Time"() -> (w1209:sgl)
        n739 = local read "Initial x (um)"() -> (w1204:dbl)
        n740 = local read "x Step (um)"() -> (w1205:dbl)
        n741 = local read "Background"() -> (w1207:i32[][])
        n742 = local read "Stage Task"() -> (w1206:refnum<k21>)
        n743 = Multiply(x=w1209, y=sgl 10.0) -> (x*y=w1208:sgl)
        n744 = stacked-sequence {
          tunnel: w1208 -> [w1227 _]
          tunnel: w1207 -> [w1226 _]
          tunnel: w1206 -> [w1225 w1307]
          tunnel: w1205 -> [w1224 _]
          tunnel: w1204 -> [w1223 _]
          tunnel: w1191 -> [w1222 _]
          tunnel: w1181 -> [w1221 _]
          tunnel: w1190 -> [w1220 w1309]
          tunnel: w1186 -> [w1219 _]
          tunnel: w1185 -> [w1218 _]
          tunnel: w1184 -> [w1217 _]
          tunnel: w1182 -> [w1216 _]
          tunnel: w1183 -> [w1215 _]
          tunnel: w1181 -> [w1214 _]
          frame #0 {
            n745 = while {
              tunnel: w1227 -> [w1246]
              tunnel: w1226 -> [w1245]
              tunnel: w1225 -> [w1243]
              tunnel: w1224 -> [w1242]
              tunnel: w1223 -> [w1241]
              shift-right: [w1239] -> _
              shift-left: w1222 -> [w1240]
              tunnel: w1221 -> [w1238]
              tunnel: w1220 -> [w1237]
              tunnel: w1219 -> [w1236]
              tunnel: w1218 -> [w1235]
              tunnel: w1217 -> [w1234]
              tunnel: w1216 -> [w1233]
              tunnel: w1215 -> [w1232]
              tunnel: w1214 -> [w1231]
              i -> [w1230]
              stop <- w1247 stop-if-true
              n746 = Multiply(x=w1242, y=w1230) -> (x*y=w1259:dbl)
              n747 = Add(x=w1259, y=w1241) -> (x+y=w1257:dbl)
              n748 = Subtract(x=w1231, y=w1230) -> (x-y=w1229:dbl)
              n749 = Divide(x=w1257, y=2.0) -> (x/y=w1254:dbl)
              n750 = call-poly <vilib>:"DAQmx Write.vi"("task/channels in"=w1243, "data"=w1254) -> ("error out"=w1258:errorcluster)  [unwired: 11 in, 2 out]
              n751 = call <userlib>:"StartAcquisition.vi"("error in (no error)"=w1258) -> ("error out"=w1255:errorcluster)  [unwired: 1 in, 1 out]
              n752 = Decrement(x=w1229) -> (x-1=w1228:dbl)
              n753 = Increment(x=w1230) -> (x+1=w1244:i32)
              n754 = while {
                tunnel: w1255 -> [_]
                tunnel: w1246 -> [w1270]
                tunnel: w1245 -> [w1269]
                tunnel: w1244 -> [w1268]
                tunnel: w1240 -> [w1267]
                tunnel: [w1266] -> w1239
                tunnel: w1228 -> [w1265]
                tunnel: w1236 -> [w1264]
                tunnel: w1235 -> [w1263]
                tunnel: w1234 -> [w1260]
                tunnel: w1233 -> [w1261]
                tunnel: w1232 -> [w1262]
                stop <- w1271 stop-if-true
                n755 = call <userlib>:"GetNumberAvailableImages.vi"() -> ("first"=w1274:i32)  [unwired: 3 in, 3 out]
                n756 = Greater Or Equal?(x=w1274, y=1) -> (x >= y?=w1272:bool)
                n757 = Wait (ms)(milliseconds to wait=w1270) -> ()  [unwired: 1 out]
                n758 = case shown="True" w1272 {
                  selector: w1272 -> [w1276 w1290]
                  tunnel: [w1276 w1290] -> w1271
                  tunnel: w1269 -> [_ w1288]
                  tunnel: w1268 -> [_ w1287]
                  tunnel: w1267 -> [w1275 w1285]
                  tunnel: [w1275 w1284] -> w1266
                  tunnel: w1265 -> [_ w1278]
                  tunnel: w1264 -> [_ w1283]
                  tunnel: w1263 -> [_ w1282]
                  tunnel: w1262 -> [_ w1281]
                  tunnel: w1261 -> [_ w1279]
                  tunnel: w1260 -> [_ w1280]
                  frame False {
                  }
                  frame True {
                    n759 = Initialize Array(w1287, w1279) -> (w1289:i32[])
                    n760 = Initialize Array(0 ("element"), w1281) -> (w1298:i32[])
                    n761 = call <userlib>:"GetMostRecentImage.vi"("size"=w1281, "array"=w1298) -> ("array"=w1296:i32[])  [unwired: 1 in, 2 out]
                    n762 = Reverse 1D Array(array=w1296) -> (reversed array=w1297:i32[])
                    n763 = Reshape Array(w1297, w1279, w1280) -> (w1295:i32[][])
                    n764 = Transpose 2D Array(2D array=w1295) -> (transposed array=w1294:i32[][])
                    n765 = Subtract(x=w1294, y=w1288) -> (x-y=w1277:i32[][])
                    n766 = Transpose 2D Array(2D array=w1277) -> (transposed array=w1291:i32[][])
                    n767 = local write "CCD Image"(w1277) -> ()
                    n768 = for {
                      tunnel: w1291 -> [w1305] mode=indexing
                      tunnel: [w1304] -> w1286 mode=indexing
                      n769 = Add Array Elements(numeric array=w1305) -> (sum=w1304:i32)
                    }
                    n770 = Build Array (concatenate)(w1289, w1277) -> (w1293:i32[][])
                    n771 = Transpose 2D Array(2D array=w1293) -> (transposed array=w1292:i32[][])
                    n772 = case shown="True" w1283 {
                      tunnel: w1292 -> [_ w1301]
                      tunnel: w1282 -> [_ w1300]
                      frame False {
                      }
                      frame True {
                        n773 = call-poly <vilib>:"Write Delimited Spreadsheet.vi"("file path (dialog if empty)"=w1300, "2D data"=w1301, "append to file? (new file:F)"=TRUE, "delimiter (\\t)"="," ("delimiter (\\t)")) -> ()  [unwired: 10 in, 2 out]
                      }
                    }
                    n774 = Replace Array Subset(array=w1285, new element=w1286, index (col)=w1278) -> (w1284:dbl[][])  [unwired: 1 in]
                    n775 = local write "Total Intensity"(w1284) -> ()
                  }
                }
              }
              n776 = Divide(x=w1244, y=w1238) -> (x/y=w1250:dbl)
              n777 = Multiply(x=w1250, y=100.0) -> (x*y=w1248:dbl)
              n778 = local write "Acquisition Progress"(w1248) -> ()
              n779 = Greater Or Equal?(x=w1244, y=w1238) -> (x >= y?=w1253:bool)
              n780 = Get Queue Status(queue=w1237) -> (# elements in queue=w1252:i32)  [unwired: 2 in, 7 out]
              n781 = Greater Than 0?(x=w1252) -> (x > 0?=w1251:bool)
              n782 = Or(x=w1251, y=w1253) -> (x .or. y?=w1247:bool)
            }
          }
          frame #1 {
            n783 = local read "Rest x (um)"() -> (w1306:dbl)
            n784 = Divide(x=w1306, y=2.0) -> (x/y=w1311:dbl)
            n785 = call-poly <vilib>:"DAQmx Write.vi"("task/channels in"=w1307, "data"=w1311) -> ("error out"=w1310:errorcluster)  [unwired: 11 in, 2 out]
            n786 = Enqueue Element(queue=w1309, element=SpectroElectroChem_1Electrode_caseEnum."Rest", error in (no error)=w1310) -> ()  [unwired: 1 in, 3 out]
          }
        }
      }
      frame "Targeted SECCM" {
        n787 = stacked-sequence {
          seq-local: [w1317 _ _ _ _] -> [_ w1359 _ _ _]
          seq-local: [w1316 _ _ _ _] -> [_ w1358 _ _ _]
          seq-local: [w1315 _ _ _ _] -> [_ w1357 _ _ _]
          seq-local: [_ w1352 _ _ _] -> [_ _ w1584 _ _]
          seq-local: [_ w1351 _ _ _] -> [_ _ _ _ _]
          seq-local: [_ w1350 _ _ _] -> [_ _ _ w1601 _]
          seq-local: [_ w1349 _ _ _] -> [_ _ _ _ w1636]
          seq-local: [_ w1348 _ _ _] -> [_ _ _ _ w1635]
          seq-local: [_ _ w1583 _ _] -> [_ _ _ w1598 _]
          seq-local: [_ _ _ w1597 _] -> [_ _ _ _ w1611]
          tunnel: w1313 -> [_ _ _ _ w1614]
          frame #0 {
            w1325 = 0.05 ("y")
            w1340 = 2.0 ("y")
            n788 = local read "CV Ef / V"() -> (w1320:dbl)
            n789 = local read "CV Ei / V"() -> (w1321:dbl)
            n790 = local read "CV v / mV/s"() -> (w1316:dbl)
            n791 = local read "CV Cycles"() -> (w1322:dbl)
            n792 = Add(x=w1320, y=w1321) -> (x+y=w1341:dbl)
            n793 = Subtract(x=w1320, y=w1321) -> (x-y=w1337:dbl)
            n794 = Absolute Value(x=w1337) -> (abs(x)=w1336:dbl)
            n795 = Multiply(x=w1336, y=1000.0) -> (x*y=w1335:dbl)
            n796 = Multiply(x=w1335, y=2.0) -> (x*y=w1332:dbl)
            n797 = Divide(x=w1316, y=w1332) -> (x/y=w1331:dbl)
            n798 = Divide(x=w1341, y=w1340) -> (x/y=w1339:dbl)
            n799 = Divide(x=w1337, y=w1340) -> (x/y=w1342:dbl)
            n800 = Divide(x=w1316, y=w1331) -> (x/y=w1330:dbl)
            n801 = Multiply(x=w1330, y=w1322) -> (x*y=w1315:dbl)
            n802 = Bundle("CV v / mV/s"=w1316, w1315) -> (w1329:cluster{"CV v / mV/s":dbl, dbl})  [unwired: 1 in]
            n803 = call <vilib>:"Triangle Waveform.vi"("offset"=w1339, "sampling info"=w1329, "reset signal"=TRUE, "phase"=270.0, "amplitude"=w1342, "frequency"=w1331) -> ("signal out"=w1328:waveform(dbl))  [unwired: 4 in, 1 out]
            n804 = Unbundle By Name(w1328) -> ("Y"=w1323:dbl[])
            n805 = Multiply(x=w1323, y=5.0) -> (x*y=w1317:dbl[])
            n806 = Max & Min(x=w1320, y=w1321) -> (max(x,y)=w1326:dbl, min(x,y)=w1327:dbl)
            n807 = Add(x=w1326, y=w1325) -> (x+y=w1319:dbl)
            n808 = Subtract(x=w1327, y=w1325) -> (x-y=w1318:dbl)
            n809 = property on="Tip Voltammogram 2" class="XYGraph (strict)"("XScale.Maximum"=w1319, "XScale.Minimum"=w1318) -> ()  [unwired: 2 in, 2 out]
          }
          frame #1 {
            n810 = local read "Points of Interest"() -> (w1366:dbl[][])
            n811 = local read "z Res. / um"() -> (w1354:dbl)
            n812 = local read "Piezo Axes"() -> (w1346:string[])
            n813 = local read "t / s/pt"() -> (w1353:dbl)
            n814 = Index Array(array=w1346, index=0) -> (element=w1361:string)
            n815 = Index Array(array=w1346, index=1) -> (element=w1360:string)
            n816 = Index Array(array=w1346, index=2) -> (element=w1362:string)
            n817 = Build Array(w1362) -> (w1352:string[])
            n818 = Divide(x=w1354, y=w1353) -> (x/y=w1351:dbl)
            n819 = Build Array(w1351) -> (w1355:dbl[])
            n820 = call "VEL.vi"("Axes to set"=w1352, "Velocity values"=w1355) -> ("error out"=w1347:errorcluster)  [unwired: 16 in, 1 out]
            n821 = Array Size(array=w1366) -> (size(s)=w1369:i32[])
            n822 = Index Array(array=w1369, index=0) -> (element=w1367:i32)
            n823 = Build Array(w1361, w1360) -> (w1350:string[])
            n824 = call "VEL?.vi"("Axes to query"=w1346, "error in"=w1347) -> ("Velocity"=w1345:dbl[], "error out"=w1344:errorcluster)  [unwired: 16 in]
            n825 = local write "Piezo Velocity / um/s"(w1345) -> ()
            n826 = while {
              tunnel: w1367 -> [w1408]
              tunnel: w1366 -> [w1406]
              tunnel: w1350 -> [w1391]
              tunnel: w1352 -> [w1402]
              tunnel: w1359 -> [w1401]
              tunnel: w1358 -> [w1400]
              tunnel: w1357 -> [w1399]
              tunnel: [w1398] -> w1349
              shift-right: [w1396] -> w1348
              shift-left: dbl[][] [] -> [w1397]
              tunnel: w1351 -> [w1395]
              tunnel: w1344 -> [w1387]
              i -> [w1393]
              stop <- w1407 stop-if-true
              w1386 = T3 0 items=["no dialog", "OK message", "continue or stop message", "OK message + warnings", "continue/stop + warnings"] ("type of dialog (OK msg:1)")
              n827 = Increment(x=w1393) -> (x+1=w1394:i32)
              n828 = Less Or Equal?(x=w1408, y=w1394) -> (x <= y?=w1407:bool)
              n829 = Index Array(array=w1406, index (row)=w1393, index (col)=0 ("disabled index (col)")) -> (element=w1385:dbl)
              n830 = Index Array(array=w1406, index (row)=w1393, index (col)=1 ("disabled index (col)")) -> (element=w1383:dbl)
              n831 = call <vilib>:"Simple Error Handler.vi"("type of dialog (OK msg:1)"=w1386, "error in (no error)"=w1387) -> ()  [unwired: 3 in, 5 out]
              n832 = local read "by"() -> (w1382:dbl)
              n833 = local read "bx"() -> (w1384:dbl)
              n834 = local read "ny"() -> (w1374:dbl)
              n835 = Subtract(x=w1385, y=w1384) -> (x-y=w1375:dbl)
              n836 = Subtract(x=w1383, y=w1382) -> (x-y=w1377:dbl)
              n837 = Multiply(x=w1375, y=w1374) -> (x*y=w1376:dbl)
              n838 = local read "nx"() -> (w1381:dbl)
              n839 = local read "dy"() -> (w1372:dbl)
              n840 = Subtract(x=w1377, y=w1376) -> (x-y=w1373:dbl)
              n841 = Multiply(x=w1381, y=w1377) -> (x*y=w1380:dbl)
              n842 = Divide(x=w1373, y=w1372) -> (x/y=w1370:dbl)
              n843 = local read "dx"() -> (w1378:dbl)
              n844 = Subtract(x=w1375, y=w1380) -> (x-y=w1379:dbl)
              n845 = Divide(x=w1379, y=w1378) -> (x/y=w1371:dbl)
              n846 = Build Array(w1371, w1370) -> (w1403:dbl[])
              n847 = call "MOV.vi"("Axes to move"=w1391, "Position values"=w1403) -> ("error out"=w1392:errorcluster)  [unwired: 17 in]
              n848 = call "General wait for movement to stop.vi"("Axes to wait for"=w1391, "All axes?"=TRUE, "error in"=w1392, "Polling cycle \ntime, ms"=u32 10 ("Polling cycle \ntime, ms")) -> ("error out"=w1388:errorcluster)  [unwired: 14 in, 1 out]
              n849 = stacked-sequence {
                seq-local: [_ _ _ _ w1435 _ _ _ _ _ _] -> [_ _ _ _ _ w1444 _ _ _ _ _]
                seq-local: [_ _ _ _ _ _ _ w1509 _ _ _] -> [_ _ _ _ _ _ _ _ w1536 _ _]
                seq-local: [_ _ _ _ _ _ _ w1508 _ _ _] -> [_ _ _ _ _ _ _ _ w1535 _ _]
                seq-local: [_ _ _ _ _ _ _ w1507 _ _ _] -> [_ _ _ _ _ _ _ _ w1533 _ _]
                seq-local: [_ _ _ _ _ _ _ _ _ w1566 _] -> [_ _ _ _ _ _ _ _ _ _ w1578]
                tunnel: w1391 -> [_ w1412 _ _ _ _ _ _ _ _ _]
                tunnel: w1402 -> [_ _ _ _ w1436 w1443 w1486 _ _ w1569 w1580]
                tunnel: [_ _ _ _ _ _ _ w1512 _ _ _] -> _
                tunnel: w1401 -> [_ _ _ _ _ _ _ w1512 _ _ _]
                tunnel: w1400 -> [_ _ _ _ _ _ _ w1514 _ _ _]
                tunnel: w1399 -> [_ _ _ _ _ _ _ w1513 w1531 _ _]
                tunnel: [_ _ _ _ _ _ _ _ w1530 _ _] -> w1398
                tunnel: [_ _ _ _ _ _ _ _ w1527 _ _] -> w1396
                tunnel: w1397 -> [_ _ _ _ _ _ _ _ w1529 _ _]
                tunnel: w1395 -> [_ _ _ _ _ _ _ _ _ _ _]
                tunnel: w1388 -> [_ _ _ _ _ _ _ _ _ _ _]
                frame #0 {
                  n850 = Wait (ms)(milliseconds to wait=u32 100) -> ()  [unwired: 1 out]
                }
                frame #1 {
                  n851 = call "POS?.vi"("Axes to query"=w1412) -> ("Position"=w1413:dbl[])  [unwired: 17 in, 1 out]
                  n852 = Index Array(array=w1413, index=1) -> (element=w1410:dbl)
                  n853 = Index Array(array=w1413, index=0) -> (element=w1411:dbl)
                  n854 = local write "Piezo x"(w1411) -> ()
                  n855 = local write "Piezo y"(w1410) -> ()
                }
                frame #2 {
                  w1426 = 10123 items=["Finite Samples"=10178, "Continuous Samples"=10123, "Hardware Timed Single Point"=12522] ("sample mode")
                  n856 = local read "Monitor"() -> (w1416:refnum<k21>)
                  n857 = local read "Econtrol"() -> (w1418:refnum<k21>)
                  n858 = local read "E Approach / V"() -> (w1417:dbl)
                  n859 = Multiply(x=w1417, y=5.0) -> (x*y=w1431:dbl)
                  n860 = Initialize Array(w1431, 2 ("dimension size")) -> (w1433:dbl[])
                  n861 = call <vilib>:"DAQmx Stop Task.vi"("task/channels in"=w1416) -> ("task out"=w1424:refnum<k21>, "error out"=w1423:errorcluster)  [unwired: 13 in]
                  n862 = call-poly <vilib>:"DAQmx Timing.vi"("task/channels in"=w1424, "sample mode"=w1426, "rate"=25000.0, "error in"=w1423) -> ("error out"=w1425:errorcluster)  [unwired: 10 in, 1 out]
                  n863 = call <vilib>:"DAQmx Stop Task.vi"("task/channels in"=w1418, "error in"=w1425) -> ("task out"=w1432:refnum<k21>, "error out"=w1428:errorcluster)  [unwired: 12 in]
                  n864 = call-poly <vilib>:"DAQmx Write.vi"("task/channels in"=w1432, "data"=w1433, "error in"=w1428) -> ("task out"=w1419:refnum<k21>, "error out"=w1421:errorcluster)  [unwired: 10 in, 1 out]
                  n865 = call-poly <vilib>:"DAQmx Trigger.vi"("task/channels in"=w1419, "error in"=w1421) -> ("task out"=w1422:refnum<k21>, "error out"=w1420:errorcluster)  [unwired: 12 in]
                  n866 = call <vilib>:"DAQmx Start Task.vi"("task/channels in"=w1422, "error in"=w1420) -> ()  [unwired: 12 in, 2 out]
                }
                frame #3 {
                  n867 = Wait (ms)(milliseconds to wait=u32 100) -> ()  [unwired: 1 out]
                }
                frame #4 {
                  n868 = local read "Monitor"() -> (w1435:refnum<k21>)
                  n869 = call "POS?.vi"("Axes to query"=w1436) -> ("Position"=w1441:dbl[], "error out"=w1439:errorcluster)  [unwired: 17 in]
                  n870 = Index Array(array=w1441, index=0) -> (element=w1437:dbl)
                  n871 = local write "Piezo z"(w1437) -> ()
                  n872 = call <vilib>:"DAQmx Start Task.vi"("task/channels in"=w1435, "error in"=w1439) -> ("error out"=w1438:errorcluster)  [unwired: 12 in, 1 out]
                  n873 = call "MOV.vi"("Axes to move"=w1436, "Position values"=dbl[] [85.0], "error in"=w1438) -> ()  [unwired: 16 in, 1 out]
                }
                frame #5 {
                  w1445 = dbl[] []
                  n874 = local read "z Res. / um"() -> (w1447:dbl)
                  n875 = local read "Piezo z"() -> (w1446:dbl)
                  n876 = while {
                    tunnel: w1447 -> [w1462]
                    tunnel: w1446 -> [w1461]
                    shift-right: [w1460] -> _
                    shift-left: w1445 -> [w1459]
                    shift-right: [w1457] -> _
                    shift-left: w1445 -> [w1456]
                    tunnel: w1444 -> [w1454]
                    tunnel: w1443 -> [w1448]
                    i -> [w1463]
                    stop <- w1449 stop-if-true
                    n877 = local read "SECCM SP Dir"() -> (w1455:u16)
                    n878 = local read "t / s/pt"() -> (w1451:dbl)
                    n879 = local read "Approach Set / A"() -> (w1452:dbl)
                    n880 = Multiply(x=w1462, y=w1463) -> (x*y=w1468:dbl)
                    n881 = local read "Tip Gain (mV/pA)"() -> (w1458:dbl)
                    n882 = Add(x=w1468, y=w1461) -> (x+y=w1450:dbl)
                    n883 = Multiply(x=w1451, y=25000.0) -> (x*y=w1469:dbl)
                    n884 = call-poly <vilib>:"DAQmx Read.vi"("task/channels in"=w1454, "number of samples per channel"=w1469) -> ("data"=w1474:dbl[][])  [unwired: 11 in, 2 out]
                    n885 = Equal?(x=w1455, y=u16 0) -> (x = y?=w1471:bool)
                    n886 = Index Array(array=w1474, index (row)=0) -> (element=w1476:dbl[])  [unwired: 1 in]
                    n887 = Multiply(x=w1458, y=1000000000.0) -> (x*y=w1465:dbl)
                    n888 = call-poly <vilib>:"Mean.vi"("X"=w1476) -> ("mean"=w1475:dbl)  [unwired: 1 out]
                    n889 = Divide(x=w1475, y=w1465) -> (x/y=w1470:dbl)
                    n890 = case shown="False" w1471 {
                      tunnel: w1452 -> [w1481 w1484]
                      tunnel: w1470 -> [w1482 w1485]
                      tunnel: [w1480 w1483] -> w1464
                      frame False {
                        n891 = Less?(x=w1482, y=w1481) -> (x < y?=w1480:bool)
                      }
                      frame True {
                        n892 = Greater?(x=w1485, y=w1484) -> (0:w1483:bool)
                      }
                    }
                    n893 = Build Array (concatenate)(w1459, w1450) -> (w1460:dbl[])
                    n894 = local write "Sample z"(w1450) -> ()
                    n895 = local write "Piezo z"(w1450) -> ()
                    n896 = Greater Or Equal?(x=w1450, y=80.0) -> (x >= y?=w1467:bool)
                    n897 = Build Array (concatenate)(w1456, w1470) -> (w1457:dbl[])
                    n898 = Bundle(w1460, w1457) -> (w1453:cluster{dbl[], dbl[]})  [unwired: 1 in]
                    n899 = local write "Tip Approach Curve 2"(w1453) -> ()
                    n900 = Or(x=w1464, y=w1467) -> (x .or. y?=w1449:bool)
                    n901 = case shown="True" w1449 {
                      tunnel: w1448 -> [_ w1479]
                      frame False {
                      }
                      frame True {
                        n902 = call "HLT.vi"("Affected axes"=w1479) -> ()  [unwired: 18 in, 1 out]
                      }
                    }
                  }
                }
                frame #6 {
                  n903 = local read "CV Ei / V"() -> (w1487:dbl)
                  n904 = local read "Monitor"() -> (w1489:refnum<k21>)
                  n905 = call "POS?.vi"("Axes to query"=w1486) -> ("Position"=w1506:dbl[])  [unwired: 17 in, 1 out]
                  n906 = local read "Econtrol"() -> (w1488:refnum<k21>)
                  n907 = call <vilib>:"DAQmx Stop Task.vi"("task/channels in"=w1489) -> ("task out"=w1493:refnum<k21>, "error out"=w1491:errorcluster)  [unwired: 13 in]
                  n908 = Multiply(x=w1487, y=5.0) -> (x*y=w1501:dbl)
                  n909 = Index Array(array=w1506, index=0) -> (element=w1490:dbl)
                  n910 = call-poly <vilib>:"DAQmx Read.vi"("task/channels in"=w1493, "timeout"=-1.0, "error in"=w1491) -> ("task out"=w1492:refnum<k21>, "error out"=w1494:errorcluster)  [unwired: 10 in, 1 out]
                  n911 = Initialize Array(w1501, 2 ("dimension size")) -> (w1504:dbl[])
                  n912 = call <vilib>:"DAQmx Stop Task.vi"("task/channels in"=w1492, "error in"=w1494) -> ("error out"=w1496:errorcluster)  [unwired: 12 in, 1 out]
                  n913 = call <vilib>:"DAQmx Stop Task.vi"("task/channels in"=w1488, "error in"=w1496) -> ("task out"=w1503:refnum<k21>, "error out"=w1498:errorcluster)  [unwired: 12 in]
                  n914 = local write "Sample z"(w1490) -> ()
                  n915 = local write "Piezo z"(w1490) -> ()
                  n916 = call-poly <vilib>:"DAQmx Write.vi"("task/channels in"=w1503, "data"=w1504, "error in"=w1498) -> ("task out"=w1502:refnum<k21>, "error out"=w1497:errorcluster)  [unwired: 10 in, 1 out]
                  n917 = call <vilib>:"DAQmx Start Task.vi"("task/channels in"=w1502, "error in"=w1497) -> ()  [unwired: 12 in, 2 out]
                }
                frame #7 {
                  w1517 = 25000.0 ("rate")
                  w1519 = 10178 items=["Finite Samples"=10178, "Continuous Samples"=10123, "Hardware Timed Single Point"=12522] ("sample mode")
                  w1520 = 10178 items=["Finite Samples"=10178, "Continuous Samples"=10123, "Hardware Timed Single Point"=12522] ("sample mode")
                  n918 = local read "Econtrol"() -> (w1510:refnum<k21>)
                  n919 = local read "Monitor"() -> (w1511:refnum<k21>)
                  n920 = call <vilib>:"DAQmx Stop Task.vi"("task/channels in"=w1510) -> ("task out"=w1523:refnum<k21>, "error out"=w1525:errorcluster)  [unwired: 13 in]
                  n921 = Divide(x=w1517, y=w1514) -> (x/y=w1507:dbl)
                  n922 = Multiply(x=w1513, y=w1507) -> (x*y=w1516:dbl)
                  n923 = call-poly <vilib>:"DAQmx Timing.vi"("task/channels in"=w1523, "sample mode"=w1520, "samples per channel"=w1513, "rate"=w1514, "error in"=w1525) -> ("task out"=w1522:refnum<k21>, "error out"=w1524:errorcluster)  [unwired: 9 in]
                  n924 = call-poly <vilib>:"DAQmx Timing.vi"("task/channels in"=w1511, "sample mode"=w1519, "samples per channel"=w1516, "rate"=w1517, "source"=tag "OnboardClock") -> ("task out"=w1508:refnum<k21>)  [unwired: 9 in, 1 out]
                  n925 = call-poly <vilib>:"DAQmx Trigger.vi"("task/channels in"=w1522, "source"=tag "/cDAQ1/ai/StartTrigger", "error in"=w1524) -> ("task out"=w1521:refnum<k21>, "error out"=w1526:errorcluster)  [unwired: 11 in]
                  n926 = call-poly <vilib>:"DAQmx Write.vi"("task/channels in"=w1521, "data"=w1512, "error in"=w1526) -> ("task out"=w1509:refnum<k21>)  [unwired: 10 in, 2 out]
                }
                frame #8 {
                  w1532 = dbl[] []
                  n927 = flat-sequence {
                    tunnel: w1536 -> [w1562]
                    tunnel: w1535 -> [w1560]
                    tunnel: [w1561] -> w1538
                    tunnel: [w1560] -> w1537
                    tunnel: w1538 -> [w1564]
                    tunnel: w1537 -> [w1565]
                    tunnel: [w1563] -> _
                    tunnel: [w1563] -> w1534
                    frame #0 {
                      n928 = call <vilib>:"DAQmx Start Task.vi"("task/channels in"=w1562) -> ("error out"=w1561:errorcluster)  [unwired: 13 in, 1 out]
                    }
                    frame #1 {
                      n929 = call <vilib>:"DAQmx Start Task.vi"("task/channels in"=w1565, "error in"=w1564) -> ("task out"=w1563:refnum<k21>)  [unwired: 12 in, 1 out]
                    }
                  }
                  n930 = while {
                    tunnel: w1534 -> [w1548]
                    tunnel: w1533 -> [w1547]
                    shift-right: [w1545] -> w1530
                    shift-left: w1532 -> [w1544]
                    shift-right: [w1543] -> w1528
                    shift-left: w1532 -> [w1542]
                    tunnel: w1531 -> [w1540]
                    stop <- w1539 stop-if-true
                    n931 = local read "Tip Gain (mV/pA)"() -> (w1546:dbl)
                    n932 = call-poly <vilib>:"DAQmx Read.vi"("task/channels in"=w1548, "number of samples per channel"=w1547) -> ("data"=w1559:dbl[][])  [unwired: 11 in, 2 out]
                    n933 = Multiply(x=w1546, y=1000000000.0) -> (x*y=w1553:dbl)
                    n934 = Index Array(array=w1559, index (row)=1) -> (element=w1555:dbl[])  [unwired: 1 in]
                    n935 = Index Array(array=w1559, index (row)=0) -> (element=w1556:dbl[])  [unwired: 1 in]
                    n936 = call-poly <vilib>:"Mean.vi"("X"=w1555) -> ("mean"=w1550:dbl)  [unwired: 1 out]
                    n937 = Build Array (concatenate)(w1544, w1550) -> (w1545:dbl[])
                    n938 = call-poly <vilib>:"Mean.vi"("X"=w1556) -> ("mean"=w1552:dbl)  [unwired: 1 out]
                    n939 = Divide(x=w1552, y=w1553) -> (x/y=w1551:dbl)
                    n940 = Build Array (concatenate)(w1542, w1551) -> (w1543:dbl[])
                    n941 = Bundle(w1545, w1543) -> (w1541:cluster{dbl[], dbl[]})  [unwired: 1 in]
                    n942 = local write "Tip Voltammogram 2"(w1541) -> ()
                    n943 = Array Size(array=w1543) -> (size(s)=w1549:i32)
                    n944 = Greater Or Equal?(x=w1549, y=w1540) -> (x >= y?=w1539:bool)
                  }
                  n945 = Build Array (concatenate)(w1529, w1528) -> (w1527:dbl[][])
                }
                frame #9 {
                  n946 = local read "Retraction / um"() -> (w1571:dbl)
                  n947 = call "POS?.vi"("Axes to query"=w1569) -> ("Position"=w1576:dbl[], "error out"=w1574:errorcluster)  [unwired: 17 in]
                  n948 = Index Array(array=w1576, index=0) -> (element=w1573:dbl)
                  n949 = Subtract(x=w1573, y=w1571) -> (x-y=w1572:dbl)
                  n950 = Build Array(w1572) -> (w1577:dbl[])
                  n951 = call "MOV.vi"("Axes to move"=w1569, "Position values"=w1577, "error in"=w1574) -> ("error out"=w1570:errorcluster)  [unwired: 16 in]
                  n952 = call "General wait for movement to stop.vi"("Axes to wait for"=w1569, "All axes?"=TRUE, "error in"=w1570, "Polling cycle \ntime, ms"=u32 10 ("Polling cycle \ntime, ms")) -> ("error out"=w1566:errorcluster)  [unwired: 14 in, 1 out]
                }
                frame #10 {
                  n953 = call "POS?.vi"("Axes to query"=w1580, "error in"=w1578) -> ("Position"=w1582:dbl[])  [unwired: 16 in, 1 out]
                  n954 = Index Array(array=w1582, index=0) -> (element=w1579:dbl)
                  n955 = local write "Sample z"(w1579) -> ()
                  n956 = local write "Piezo z"(w1579) -> ()
                }
              }
            }
          }
          frame #2 {
            n957 = call "POS?.vi"("Axes to query"=w1584) -> ("Position"=w1594:dbl[], "error out"=w1595:errorcluster)  [unwired: 17 in]
            n958 = Index Array(array=w1594, index=0) -> (element=w1589:dbl)
            n959 = Subtract(x=w1589, y=5.0) -> (x-y=w1591:dbl)
            n960 = Max & Min(x=w1591, y=0.0) -> (max(x,y)=w1588:dbl)  [unwired: 1 out]
            n961 = Build Array(w1588) -> (w1596:dbl[])
            n962 = local write "Sample z"(w1588) -> ()
            n963 = call "MOV.vi"("Axes to move"=w1584, "Position values"=w1596, "error in"=w1595) -> ("error out"=w1587:errorcluster)  [unwired: 16 in]
            n964 = call "General wait for movement to stop.vi"("Axes to wait for"=w1584, "All axes?"=TRUE, "error in"=w1587, "Polling cycle \ntime, ms"=u32 10 ("Polling cycle \ntime, ms")) -> ("error out"=w1583:errorcluster)  [unwired: 14 in, 1 out]
          }
          frame #3 {
            w1603 = 0.0 ("element")
            n965 = local write "Sample x"(w1603) -> ()
            n966 = local write "Sample y"(w1603) -> ()
            n967 = Build Array(w1603, w1603) -> (w1604:dbl[])
            n968 = call "MOV.vi"("Axes to move"=w1601, "Position values"=w1604, "error in"=w1598) -> ("error out"=w1602:errorcluster)  [unwired: 16 in]
            n969 = call "General wait for movement to stop.vi"("Axes to wait for"=w1601, "All axes?"=TRUE, "error in"=w1602, "Polling cycle \ntime, ms"=u32 10 ("Polling cycle \ntime, ms")) -> ("error out"=w1597:errorcluster)  [unwired: 14 in, 1 out]
          }
          frame #4 {
            w1605 = T3 0 items=["no dialog", "OK message", "continue or stop message", "OK message + warnings", "continue/stop + warnings"] ("type of dialog (OK msg:1)")
            w1620 = 10123 items=["Finite Samples"=10178, "Continuous Samples"=10123, "Hardware Timed Single Point"=12522] ("sample mode")
            n970 = Two Button Dialog(message="Save CV Data?", 1:"No" ("F button name (\"Cancel\")"), 2:"Yes" ("T button name (\"OK\")")) -> (T button?=w1640:bool)
            n971 = Enqueue Element(queue=w1614, element=SpectroElectroChem_1Electrode_caseEnum."Rest") -> ()  [unwired: 2 in, 3 out]
            n972 = local read "Piezo Axes"() -> (w1608:string[])
            n973 = call "POS?.vi"("Axes to query"=w1608, "error in"=w1611) -> ("Position"=w1647:dbl[], "error out"=w1610:errorcluster)  [unwired: 16 in]
            n974 = Index Array(array=w1647, index=1) -> (element=w1642:dbl)
            n975 = Index Array(array=w1647, index=0) -> (element=w1643:dbl)
            n976 = Index Array(array=w1647, index=2) -> (element=w1641:dbl)
            n977 = local write "Piezo x"(w1643) -> ()
            n978 = local write "Piezo z"(w1641) -> ()
            n979 = local write "Piezo y"(w1642) -> ()
            n980 = local read "WE Rest E (V)"() -> (w1615:dbl)
            n981 = call "VEL.vi"("Axes to set"=w1608, "Velocity values"=dbl[] [100.0, 100.0, 100.0], "error in"=w1610) -> ("error out"=w1609:errorcluster)  [unwired: 15 in, 1 out]
            n982 = call "VEL?.vi"("Axes to query"=w1608, "error in"=w1609) -> ("Velocity"=w1612:dbl[], "error out"=w1606:errorcluster)  [unwired: 16 in]
            n983 = local read "Econtrol"() -> (w1616:refnum<k21>)
            n984 = Multiply(x=w1615, y=5.0) -> (x*y=w1624:dbl)
            n985 = Initialize Array(w1624, 2 ("dimension size")) -> (w1622:dbl[])
            n986 = local write "Piezo Velocity / um/s"(w1612) -> ()
            n987 = call <vilib>:"DAQmx Stop Task.vi"("task/channels in"=w1616) -> ("task out"=w1623:refnum<k21>, "error out"=w1627:errorcluster)  [unwired: 13 in]
            n988 = call <vilib>:"Simple Error Handler.vi"("type of dialog (OK msg:1)"=w1605, "error in (no error)"=w1606) -> ()  [unwired: 3 in, 5 out]
            n989 = local read "Monitor"() -> (w1617:refnum<k21>)
            n990 = call-poly <vilib>:"DAQmx Write.vi"("task/channels in"=w1623, "data"=w1622, "error in"=w1627) -> ("task out"=w1628:refnum<k21>, "error out"=w1629:errorcluster)  [unwired: 10 in, 1 out]
            n991 = call-poly <vilib>:"DAQmx Trigger.vi"("task/channels in"=w1628, "error in"=w1629) -> ("task out"=w1631:refnum<k21>, "error out"=w1630:errorcluster)  [unwired: 12 in]
            n992 = call <vilib>:"DAQmx Stop Task.vi"("task/channels in"=w1617) -> ("task out"=w1618:refnum<k21>)  [unwired: 13 in, 1 out]
            n993 = Build Array (concatenate)(w1636, w1635) -> (w1634:dbl[][])
            n994 = call <vilib>:"DAQmx Start Task.vi"("task/channels in"=w1631, "error in"=w1630) -> ("error out"=w1632:errorcluster)  [unwired: 12 in, 1 out]
            n995 = Transpose 2D Array(2D array=w1634) -> (transposed array=w1633:dbl[][])
            n996 = case shown="True" w1640 {
              tunnel: w1633 -> [_ w1660]
              frame False {
              }
              frame True {
                n997 = call-poly <vilib>:"Write Delimited Spreadsheet.vi"("format (%.3f)"="%.3e", "2D data"=w1660) -> ("new file path (Not A Path if cancelled)"=w1659:path)  [unwired: 12 in, 1 out]
                n998 = Strip Path(path=w1659) -> (stripped path=w1651:path, name=w1658:string)
                n999 = String Length(string=w1658) -> (length=w1656:i32)
                n1000 = Subtract(x=w1656, y=0) -> (x-y=w1657:i32)
                n1001 = String Subset(string=w1658, length (rest)=w1657) -> (substring=w1654:string)  [unwired: 1 in]
                n1002 = local read "Points of Interest"() -> (w1648:dbl[][])
                n1003 = Concatenate Strings(w1654, "_POI" ("string")) -> (w1652:string)
                n1004 = Build Path(base path=w1651, name or relative path=w1652) -> (appended path=w1650:path)
                n1005 = call-poly <vilib>:"Write Delimited Spreadsheet.vi"("file path (dialog if empty)"=w1650, "format (%.3f)"="%.3e", "2D data"=w1648) -> ()  [unwired: 11 in, 2 out]
              }
            }
            n1006 = call-poly <vilib>:"DAQmx Timing.vi"("task/channels in"=w1618, "sample mode"=w1620, "rate"=25000.0, "source"=tag "OnboardClock", "error in"=w1632) -> ()  [unwired: 9 in, 2 out]
          }
        }
      }
    }
  }
  n1007 = while {
    tunnel: w6 -> [w1662]
    stop <- w1663 stop-if-true
    n1008 = event shown="[18] \"x\", \"x'\", \"y'\", \"y\": Value Change" {
      selector: _ -> [_ _ _ _ _ _ _ _ _ _ _ _ _ _ _ _ _ _ _]
      dyn-events: _ -> [_ _ _ _ _ _ _ _ _ _ _ _ _ _ _ _ _ _ _]
      timeout: _ -> [_ _ _ _ _ _ _ _ _ _ _ _ _ _ _ _ _ _ _]
      tunnel: [_ _ TRUE _ _ _ _ _ _ _ _ _ _ _ _ _ _ _ _] -> w1663
      tunnel: w1662 -> [_ w1665 w1667 w1670 w1672 w1675 w1678 w1680 w1683 w1685 w1686 w1689 w1690 w1693 w1695 w1697 _ _ _]
      event Timeout {
        n1009 = event-data() -> ()  [unwired: 1 in, 3 out]
      }
      event "Stop Action": Value Change {
        n1010 = event-data() -> ()  [unwired: 1 in, 6 out]
        n1011 = Enqueue Element(queue=w1665, element=SpectroElectroChem_1Electrode_caseEnum."Rest") -> ()  [unwired: 2 in, 3 out]
      }
      event "Shutdown": Value Change {
        n1012 = event-data() -> ()  [unwired: 1 in, 6 out]
        n1013 = Enqueue Element(queue=w1667, element=SpectroElectroChem_1Electrode_caseEnum."Shutdown") -> ()  [unwired: 2 in, 3 out]
      }
      event "Sample x", "Sample y", "Sample z": Value Change {
        n1014 = event-data() -> ()  [unwired: 1 in, 6 out]
        n1015 = Enqueue Element(queue=w1670, element=SpectroElectroChem_1Electrode_caseEnum."Move Piezo") -> ()  [unwired: 2 in, 3 out]
      }
      event "HSS (MHz)", "VSS (us)", "Binning", "EM Gain", "# of Acc.", "Exp. Time": Value Change {
        n1016 = event-data() -> ()  [unwired: 1 in, 6 out]
        n1017 = Enqueue Element(queue=w1672, element=SpectroElectroChem_1Electrode_caseEnum."Setup CCD") -> ()  [unwired: 2 in, 3 out]
      }
      event "Grating": Value Change {
        n1018 = event-data() -> ()  [unwired: 1 in, 6 out]
        n1019 = Enqueue Element(queue=w1675, element=SpectroElectroChem_1Electrode_caseEnum."Change Grating") -> ()  [unwired: 2 in, 3 out]
        n1020 = property on="Acquisition Progress" class="Slide (strict)"("Value"=u8 50 ("Acquisition Progress")) -> ()  [unwired: 2 in, 2 out]
      }
      event "Center Wavelength (nm)": Value Change {
        n1021 = event-data() -> ()  [unwired: 1 in, 6 out]
        n1022 = Enqueue Element(queue=w1678, element=SpectroElectroChem_1Electrode_caseEnum."Move Grating") -> ()  [unwired: 2 in, 3 out]
        n1023 = property on="Acquisition Progress" class="Slide (strict)"("Value"=u8 50 ("Acquisition Progress")) -> ()  [unwired: 2 in, 2 out]
      }
      event "Slit Width (um)": Value Change {
        n1024 = event-data() -> ()  [unwired: 1 in, 6 out]
        n1025 = Enqueue Element(queue=w1680, element=SpectroElectroChem_1Electrode_caseEnum."Adjust Slit") -> ()  [unwired: 2 in, 3 out]
        n1026 = property on="Acquisition Progress" class="Slide (strict)"("Value"=u8 50 ("Acquisition Progress")) -> ()  [unwired: 2 in, 2 out]
      }
      event "Aquire Background": Value Change {
        n1027 = event-data() -> ()  [unwired: 1 in, 6 out]
        n1028 = Enqueue Element(queue=w1683, element=SpectroElectroChem_1Electrode_caseEnum."Acquire CCD BG") -> ()  [unwired: 2 in, 3 out]
      }
      event "Clear Background": Value Change {
        n1029 = event-data() -> ()  [unwired: 1 in, 6 out]
        n1030 = Enqueue Element(queue=w1685, element=SpectroElectroChem_1Electrode_caseEnum."Clear CCD BG") -> ()  [unwired: 2 in, 3 out]
      }
      event "WE Rest E (V)": Value Change {
        n1031 = event-data() -> ()  [unwired: 1 in, 6 out]
        n1032 = Enqueue Element(queue=w1686, element=SpectroElectroChem_1Electrode_caseEnum."Set E") -> ()  [unwired: 2 in, 3 out]
      }
      event "Get HSI": Value Change {
        n1033 = event-data() -> ()  [unwired: 1 in, 6 out]
        n1034 = Enqueue Element(queue=w1689, element=SpectroElectroChem_1Electrode_caseEnum."Acquire HSI") -> ()  [unwired: 2 in, 3 out]
      }
      event "Start CV": Value Change {
        n1035 = event-data() -> ()  [unwired: 1 in, 6 out]
        n1036 = Enqueue Element(queue=w1690, element=SpectroElectroChem_1Electrode_caseEnum."Acquire CV") -> ()  [unwired: 2 in, 3 out]
      }
      event "Start Approach Curve": Value Change {
        n1037 = event-data() -> ()  [unwired: 1 in, 6 out]
        n1038 = Enqueue Element(queue=w1693, element=SpectroElectroChem_1Electrode_caseEnum."Approach Curve") -> ()  [unwired: 2 in, 3 out]
      }
      event "Start SECM Image": Value Change {
        n1039 = event-data() -> ()  [unwired: 1 in, 6 out]
        n1040 = Enqueue Element(queue=w1695, element=SpectroElectroChem_1Electrode_caseEnum."Acquire SECCM Image") -> ()  [unwired: 2 in, 3 out]
      }
      event "Targeted SECCM": Value Change {
        n1041 = event-data() -> ()  [unwired: 1 in, 6 out]
        n1042 = Enqueue Element(queue=w1697, element=SpectroElectroChem_1Electrode_caseEnum."Targeted SECCM") -> ()  [unwired: 2 in, 3 out]
      }
      event "Total Intensity": Mouse Down {
        n1043 = event-data() -> ("Coords"=w1702:T4)  [unwired: 1 in, 7 out]
        n1044 = invoke on="Total Intensity" class="IntGraph (strict)" method="Map Coords To XY"("Coords"=w1702) -> ("XY"=w1701:cluster{"X":dbl, "Y":dbl})  [unwired: 6 in, 6 out]
        n1045 = local read "Points of Interest"() -> (w1698:dbl[][])
        n1046 = Cluster To Array(cluster=w1701) -> (array=w1700:dbl[])
        n1047 = Build Array (concatenate)(w1698, w1700) -> (w1699:dbl[][])
        n1048 = local write "Points of Interest"(w1699) -> ()
      }
      event "Clear POI": Value Change {
        n1049 = event-data() -> ()  [unwired: 1 in, 6 out]
        n1050 = Initialize Array(0.0 ("element"), 0 ("dimension size"), 2 ("dimension size")) -> (w1703:dbl[][])
        n1051 = local write "Points of Interest"(w1703) -> ()
      }
      event "x", "x'", "y'", "y": Value Change {
        n1052 = event-data() -> ()  [unwired: 1 in, 6 out]
        n1053 = Subtract(x="x'", y="x") -> (x-y=→"bx":dbl)
        n1054 = Subtract(x="y'", y="y") -> (x-y=→"by":dbl)
        n1055 = Divide(x="Beta", y="Alpha") -> (x/y=w1710:dbl)
        "ny" <- w1710
        n1056 = Multiply(x=w1710, y="Gamma") -> (x*y=w1708:dbl)
        n1057 = Divide(x="Gamma", y="Delta") -> (x/y=w1716:dbl)
        "nx" <- w1716
        n1058 = Subtract(x="Delta", y=w1708) -> (x-y=→"dy":dbl)
        n1059 = Multiply(x="Beta", y=w1716) -> (x*y=w1715:dbl)
        n1060 = Subtract(x="Alpha", y=w1715) -> (x-y=→"dx":dbl)
      }
    }
  }
